vi "Gestione sensori.vi"() -> ()   [LabVIEW 2019]
uses:
  <vilib>/Utility/miscctls.llb/LVRowAndColumnTypeDef.ctl
  <vilib>/Analysis/6fits.llb/Curve Fitting Criteria.ctl
  BenchSelector.vi
  <vilib>/Utility/file.llb/Read Delimited Spreadsheet (string).vi
  Global ingressi analogici.vi
  <vilib>/Analysis/polynomials.llb/Polynomial Plot (Range).vi
  <vilib>/Analysis/1siggen.llb/Ramp Pattern by Delta.vi
  <vilib>/Utility/file.llb/Write Delimited Spreadsheet (string).vi
  <vilib>/Analysis/NI_AALPro.lvlib
  <vilib>/gmath/NI_Gmath.lvlib
  <vilib>/Analysis/NI_AALBase.lvlib
panel:
  out "Row":i32
  out "Input":string[][](array[string])
  out "riga sensore da modificare":string
  out "nome e desc sensore da modificare":string
  out "all rows":string[][](array[string])
  in  "LISTA SENSORI ASSOCIATI":i32(listbox)
  out "Edit Position":T1
  in  "stop":bool
  in  "Unità di Misura":T2
  in  "Tab Control":T3(tab)
  in  "Salva modifica sensore":bool
  in  "SENSORE SELEZIONATO":T4
  in  "modifica sensore":bool
  in  "aggiungi nuovo sensore":bool
  in  "NUOVO SENSORE":T4 {"AI_max" min=0.0}
  in  "carica lista sensori":bool
  in  "Salva lista sensori":bool
  in  "ELIMINA SENSORE":bool
  in  "LISTA SENSORI 2":i32(listbox) caption="LISTA SENSORI"
  in  "MANAGER FUNZIONE CORRETTRICE":bool
  out "MASCHERA 2":bool
  in  "Cluster Funzione correttrice":T5 caption="MANAGER FUNZIONI CORRETTRICI PER LA CATENA INGRESSO+SENSORE"
  out "MASCHERA":bool
  in  "carica mappatura":bool
  in  "Salva mappatura ingressi sensori":bool
  in  "Elimina sensori ingresso selezionato":bool
  in  "Associa sensore":bool
  in  "LISTA SENSORI":i32(listbox) caption="LISTA SENSORI DISPONIBILI"
  in  "MAPPATURA":string[][](table)
  in  "LISTA INGRESSI 3":i32(listbox) caption="LISTA INGRESSI IMPIANTO"
  in  "elimina riga 25":bool
  in  "elimina riga 24":bool
  in  "elimina riga 23":bool
  in  "elimina riga 22":bool
  in  "elimina riga 21":bool
  in  "LINEA 5 - COPPIA":i32(listbox)
  in  "LINEA 4 - COPPIA":i32(listbox)
  in  "LINEA 3 - COPPIA":i32(listbox)
  in  "LINEA 2 - COPPIA":i32(listbox)
  in  "LINEA 1 - COPPIA":i32(listbox)
  in  "elimina riga 20":bool
  in  "elimina riga 19":bool
  in  "elimina riga 18":bool
  in  "elimina riga 17":bool
  in  "elimina riga 16":bool
  in  "LINEA 5 - PRESSIONE PREMISTOPPA":i32(listbox)
  in  "LINEA 4 - PRESSIONE PREMISTOPPA":i32(listbox)
  in  "LINEA 3 - PRESSIONE PREMISTOPPA":i32(listbox)
  in  "LINEA 2 - PRESSIONE PREMISTOPPA":i32(listbox)
  in  "LINEA 1 - PRESSIONE PREMISTOPPA":i32(listbox)
  in  "elimina riga 15":bool
  in  "elimina riga 14":bool
  in  "elimina riga 13":bool
  in  "elimina riga 12":bool
  in  "elimina riga 11":bool
  in  "elimina riga 10":bool
  in  "elimina riga 9":bool
  in  "elimina riga 8":bool
  in  "elimina riga 7":bool
  in  "elimina riga 6":bool
  in  "elimina riga 5":bool
  in  "elimina riga 4":bool
  in  "elimina riga 3":bool
  in  "elimina riga 2":bool
  in  "SVUOTA TUTTO MAPPATURA":bool
  in  "LINEA 5 - PORTATA":i32(listbox)
  in  "LINEA 5 - PRESSIONE ASPIRAZIONE":i32(listbox)
  in  "LINEA 5 - PRESSIONE MANDATA":i32(listbox)
  in  "LINEA 4 - PORTATA":i32(listbox)
  in  "LINEA 4 - PRESSIONE ASPIRAZIONE":i32(listbox)
  in  "LINEA 4 - PRESSIONE MANDATA":i32(listbox)
  in  "carica assoc ingressi- linee":bool
  in  "SALVA ASSOC INGRESSI-LINEE":bool
  in  "LINEA 3 - PORTATA":i32(listbox)
  in  "LINEA 3 - PRESSIONE ASPIRAZIONE":i32(listbox)
  in  "LINEA 3 - PRESSIONE MANDATA":i32(listbox)
  in  "LINEA 2 - PORTATA":i32(listbox)
  in  "LINEA 2 - PRESSIONE ASPIRAZIONE":i32(listbox)
  in  "LINEA 2 - PRESSIONE MANDATA":i32(listbox)
  in  "LINEA 1 - PORTATA":i32(listbox)
  in  "LINEA 1 - PRESSIONE ASPIRAZIONE":i32(listbox)
  in  "LINEA 1 - PRESSIONE MANDATA":i32(listbox)
  in  "LISTA INGRESSI 2":i32(listbox) caption="LISTA INGRESSI"
  in  "elimina riga 1":bool
  in  "Tree":string(tree)
  in  "Cancel Button 2":bool
  in  "Cancel Button":bool
  in  "ASSOCIA 2":bool
  in  "Lista ingressi":i32(listbox)
  in  "ASSOCIA":bool
  in  "Sensori associabili all'ingresso selezionato":i32(listbox)
  # "CLICCA E DIGITA NELLA CELLA DI INTERESSE\nPER IMPOSTARE I VALORI DESIDERATI\nDI RANGE/OFFSET/UM"
  # "CLICCA PER SELEZIONARE \nLA RIGA DI INTERESSE"
  # "MODALITA' DI CONVERSIONE UTILIZZATA PER\nL'INGRESSO+SENSORE SELEZIONATO"
  # "1-SELEZIONA L'INGRESSO DELL'IMPIANTO DESIDERATO DALLA TABELLA \"LISTA INGRESSI IMPIANTO\"\n2-SELEZIONARE IL SENSORE CHE SI VUOLE ASSOCIARE ALL'INGRESSO DALLA TABELLA \"LISTA SENSORI DISPONIBILI\"\n3-CLICCARE \"ASSOCIA SENSORE\"\n4-INSERIRE UM, RANGE ED OFFSET (RELATIVO ALLA CATENA INGRESSO-SENSORE) NELLA TABELLA AFFIANCO\n5-SALVARE LA MAPPATURA CLICCANDO \"SALVA MAPPATURA\""
  # "Inserisci il valore fisico\nimpostato dallo strumento\ndi riferimento"
  # "0=linear fit"
  # "LINEA 1 - VASCA"
  # "LINEA 1 - SERBATOIO"
  # "LINEA 2 - SERBATOIO"
  # "LINEA 3 - SERBATOIO"
  # "LINEA 2 - VASCA"
  # "CLICCA L'INGRESSO DI INTERESSE NELLA \"LISTA INGRESSI\"\nE TRASCINALO NELLA TABELLA OPPORTUNA"
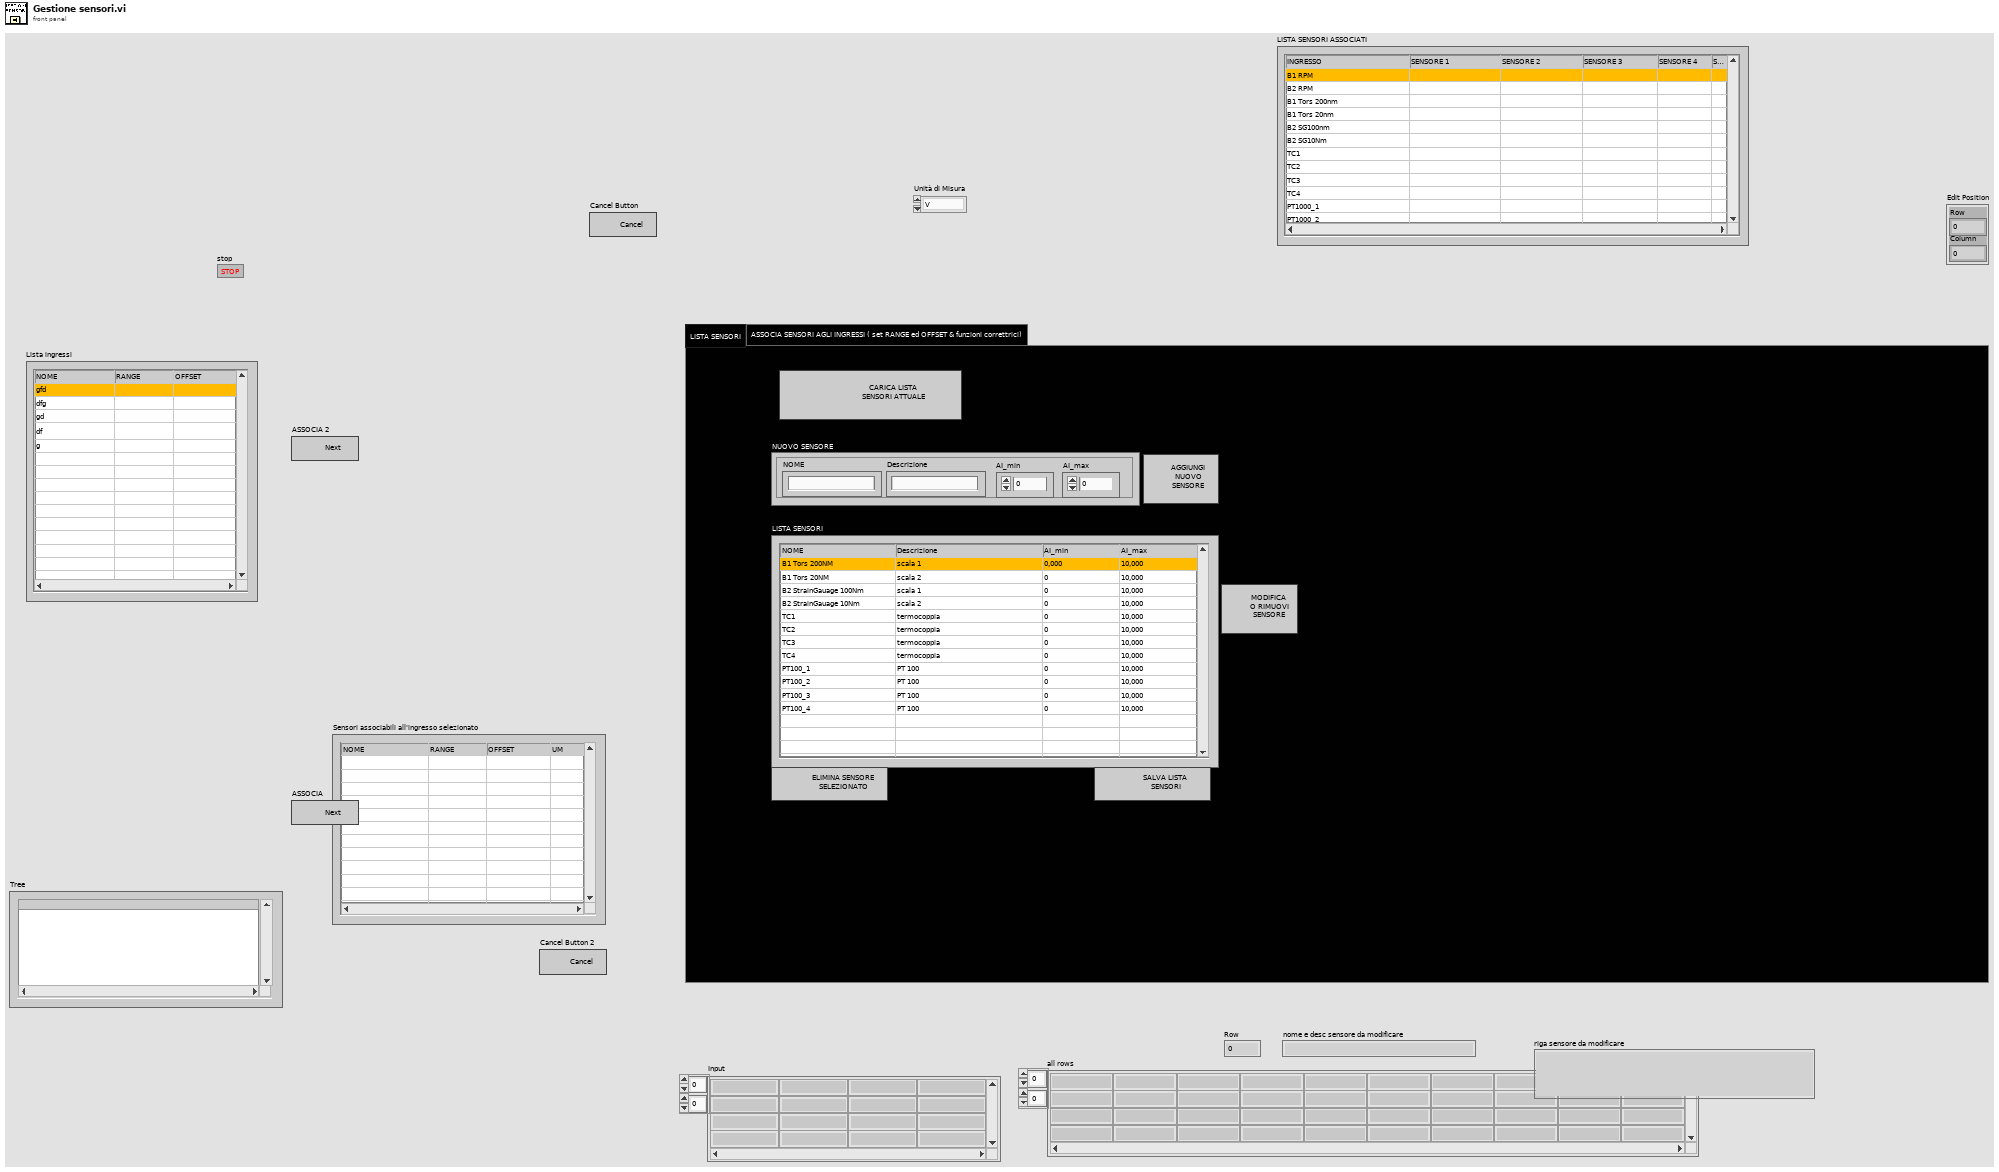
[diagram p1: front panel]
types:
  T1 = typedef "LVRowAndColumnTypeDef.ctl" = cluster{"Row":i32, "Column":i32}
  T2 = typedef "UnitàMisura.ctl" = enum16{"V", "mA", "Bar", "RPM", "m3/s", "m3/min", "m3/h", "l/s", "l/min", "in3/min", "ft3/min", "gpm", "igpm", "igph", "%", "°C", "m", "Nm", "A"}
  T3 = enum32{"LISTA SENSORI", "ASSOCIA SENSORI AGLI INGRESSI ( set RANGE ed OFFSET & funzioni correttrici)", "ASSOCIA GLI INGRESSI ALLE LINEE IDRAULICHE"}
  T4 = cluster{"NOME":string, "Descrizione":string, "AI_min":dbl, "AI_max":dbl}
  T5 = cluster{"Ingresso analogico":dbl, "NOME INGRESSO":string, "NOME SENSORE":string, "DESCRIZIONE":string, "PUNTI FUNZIONE CORRETTRICE":i32, "VALORE FISICO":dbl, "ACQUISISCI PUNTO":bool, "ELIMINA PUNTO":bool, "Valore ingresso analogico":enum32{"Leggi dal campo", "Imposta manualmente"}, "salva funzione correttrice":bool, "Ordine polinomio fit":i16, "Graph":cluster{"Ramp Pattern":dbl[], "P(A)":dbl[]}[], "UM":string, "CHIUDI":bool, "USA FUNZIONE CORRETTRICE?":bool}
  T6 = enum8{"Enabled", "Disabled", "Disabled and Grayed Out"}
  T7 = typedef "NI_AALPro.lvlib/Curve Fitting Criteria.ctl" = u16
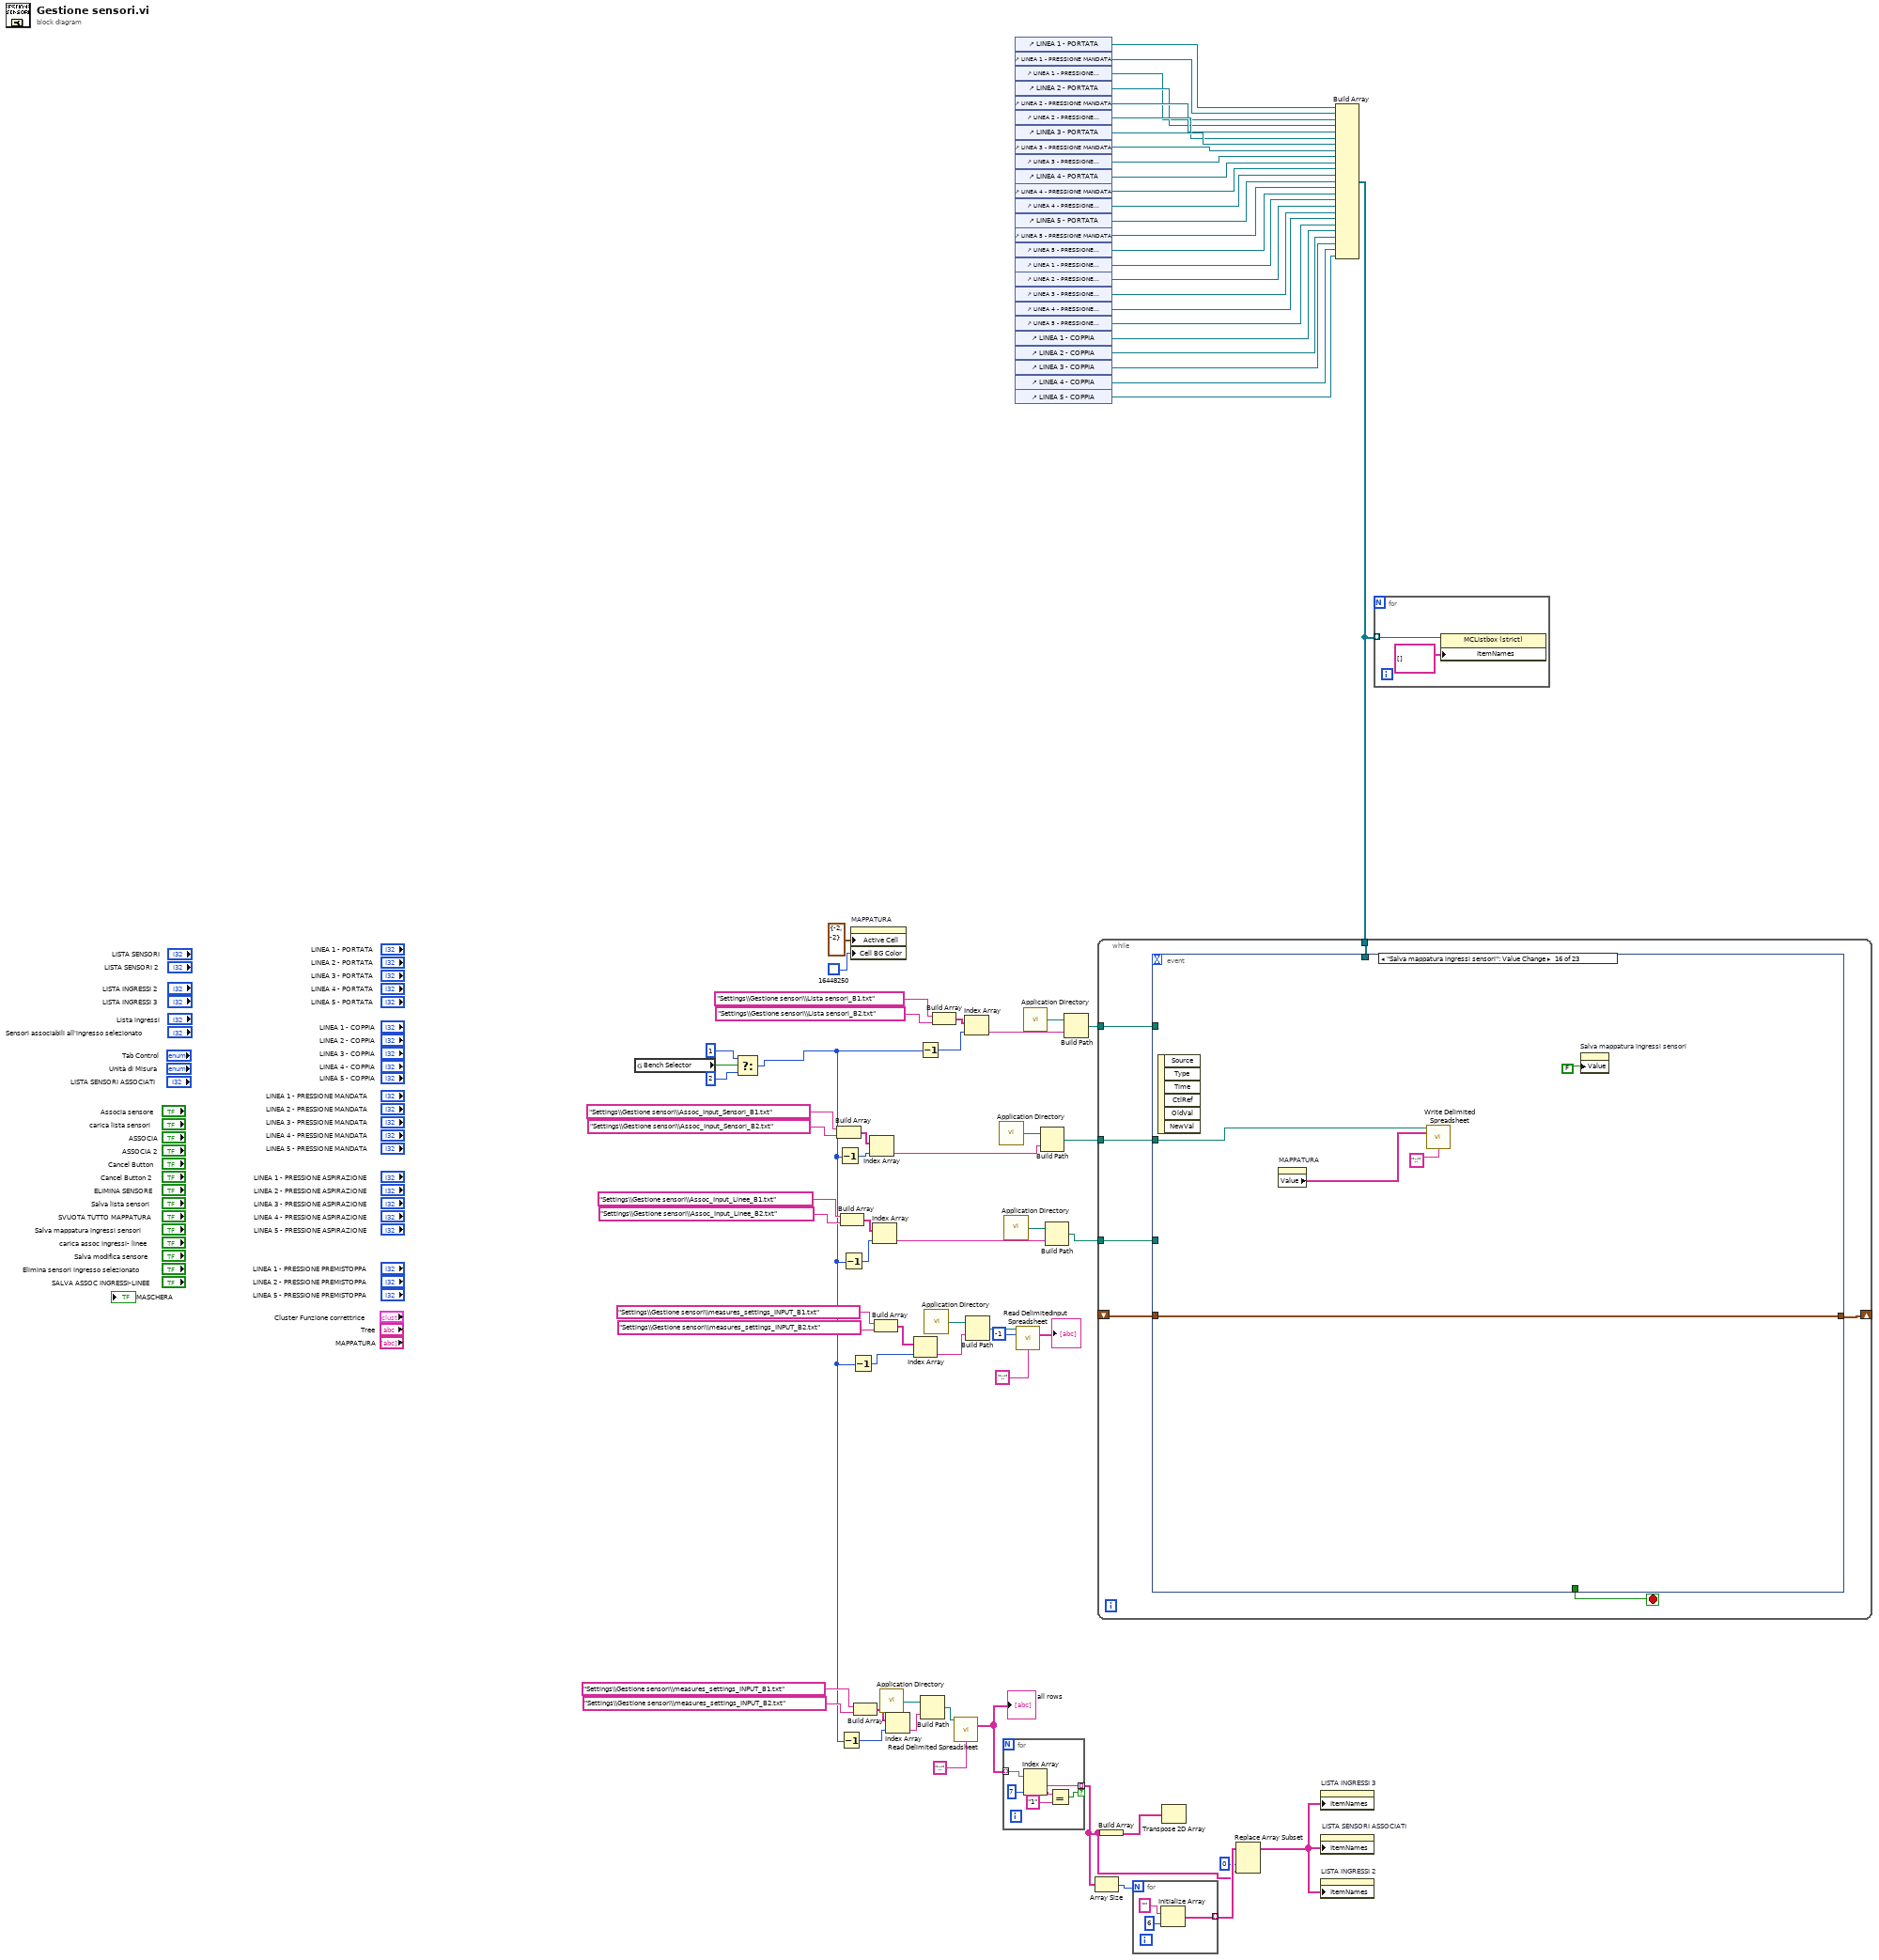
[diagram p0: block diagram]
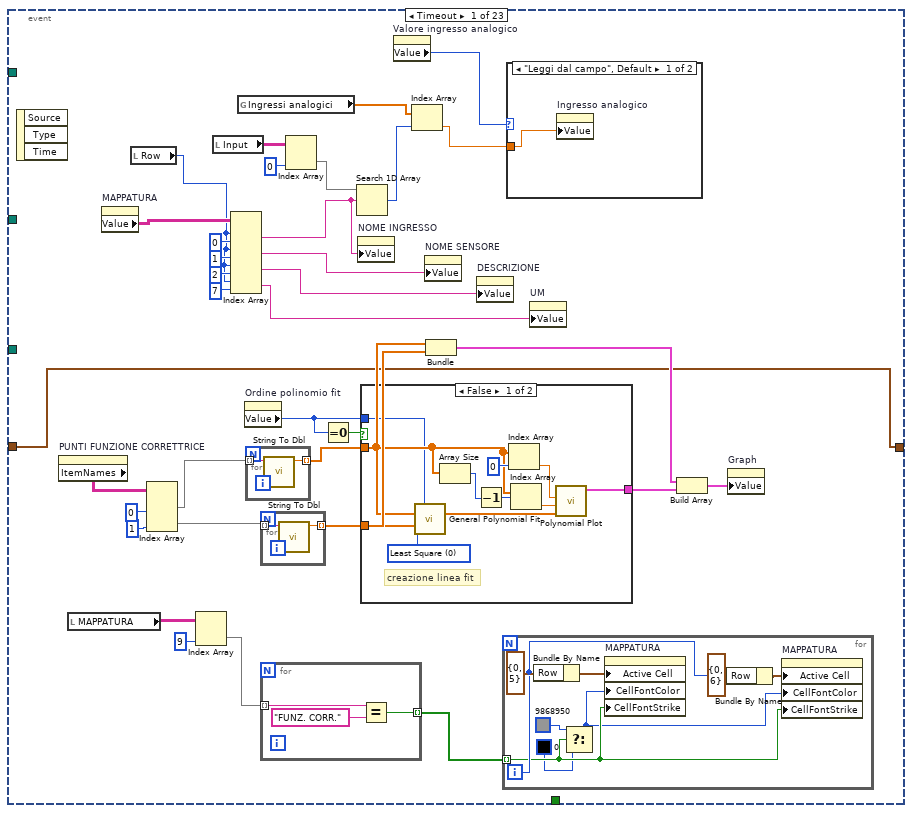
[diagram p2: hidden frame]
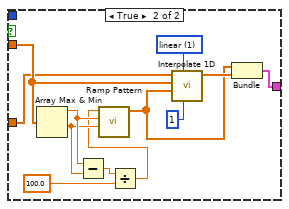
[diagram p3: hidden frame]
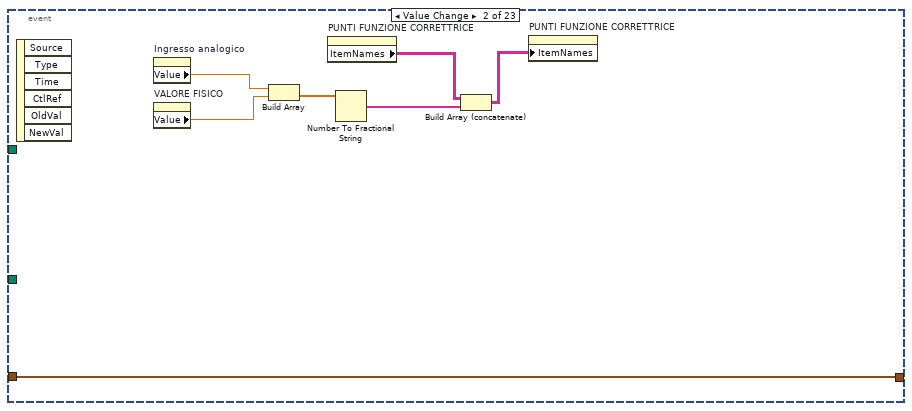
[diagram p5: hidden frame]
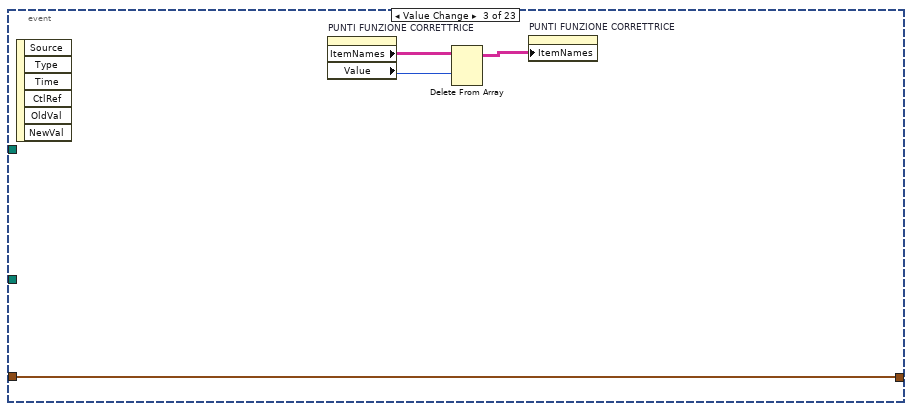
[diagram p6: hidden frame]
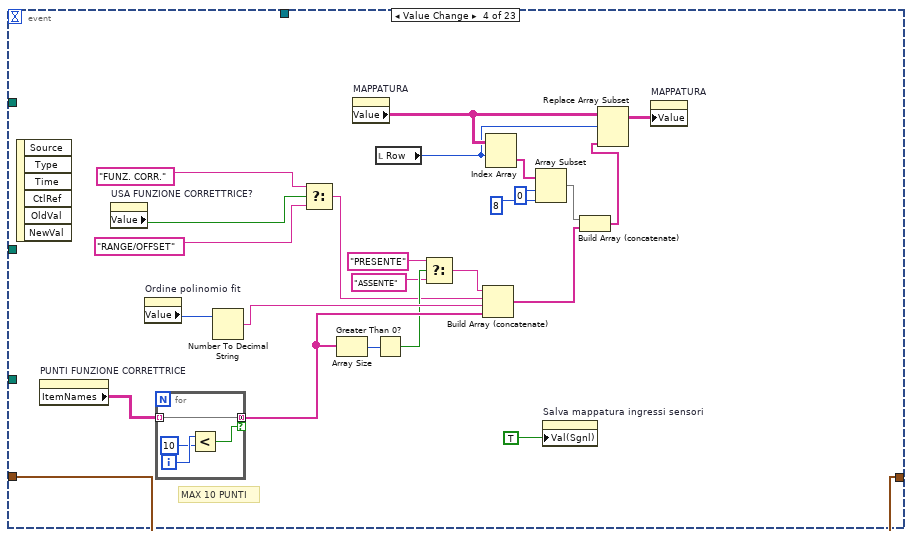
[diagram p7: hidden frame]
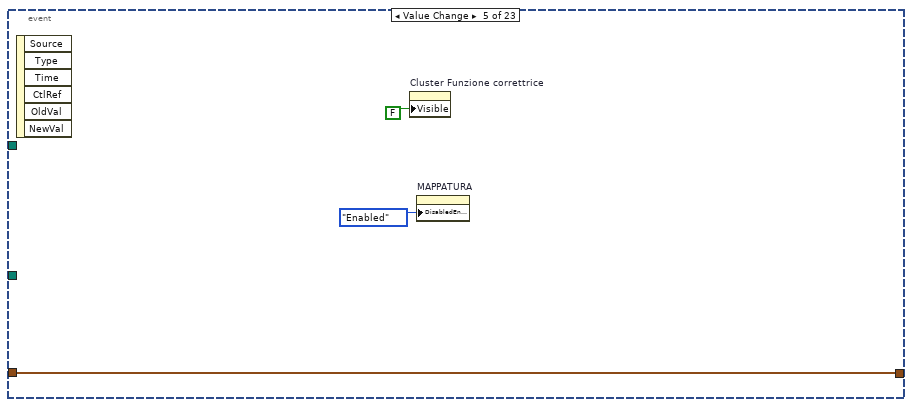
[diagram p8: hidden frame]
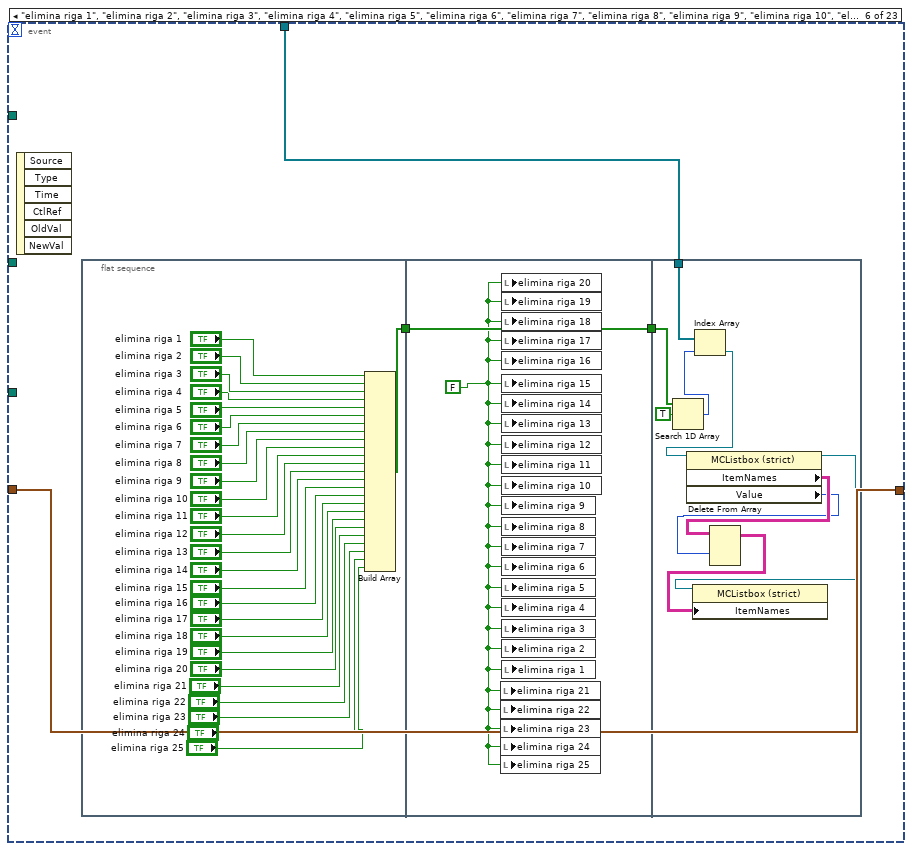
[diagram p9: hidden frame]
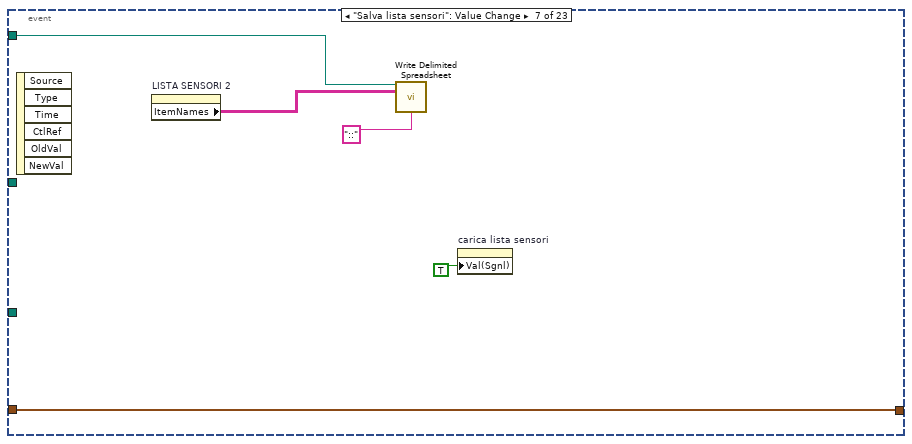
[diagram p10: hidden frame]
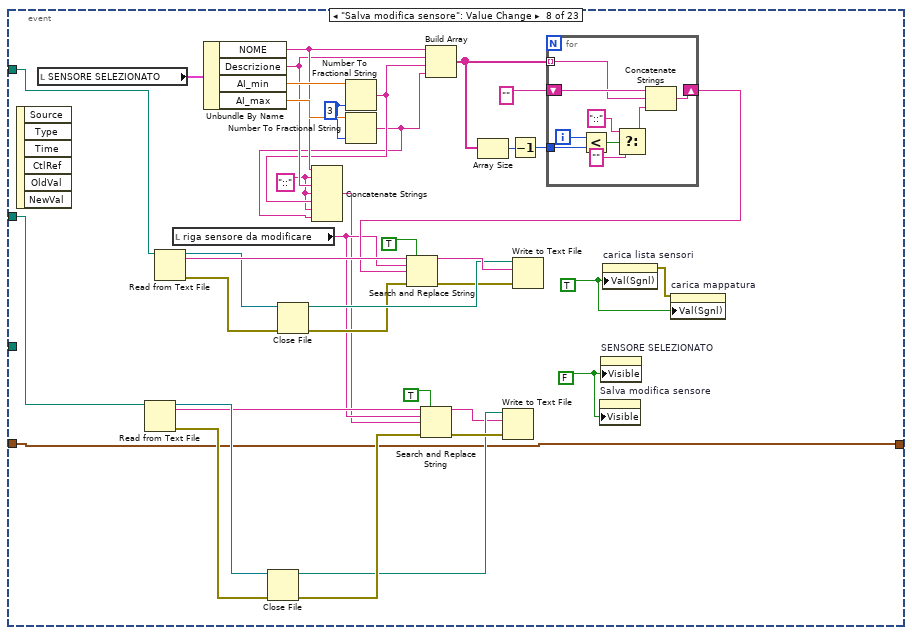
[diagram p11: hidden frame]
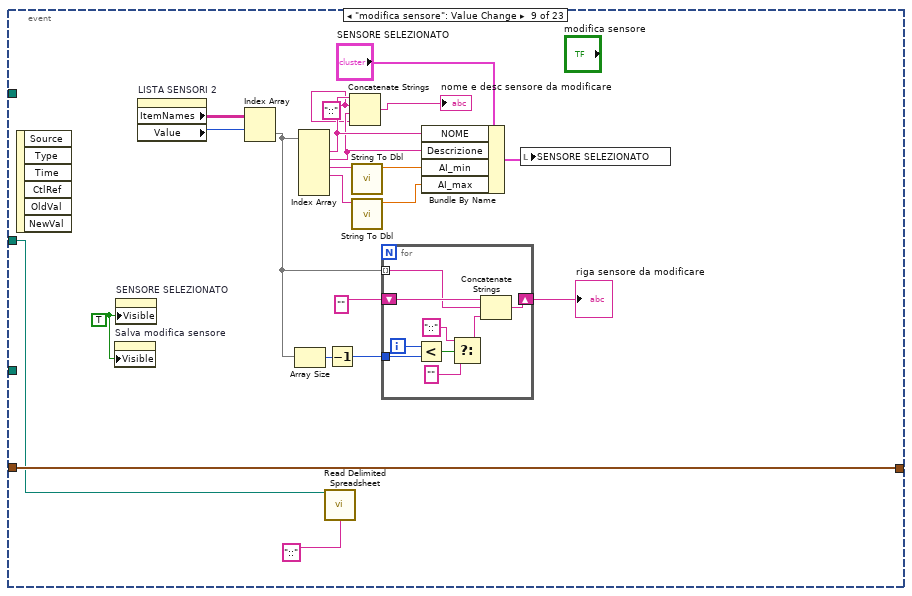
[diagram p12: hidden frame]
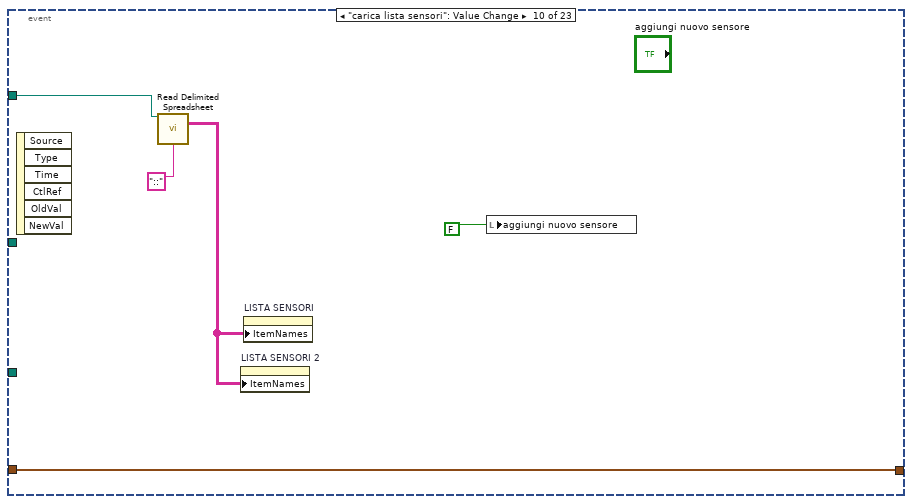
[diagram p13: hidden frame]
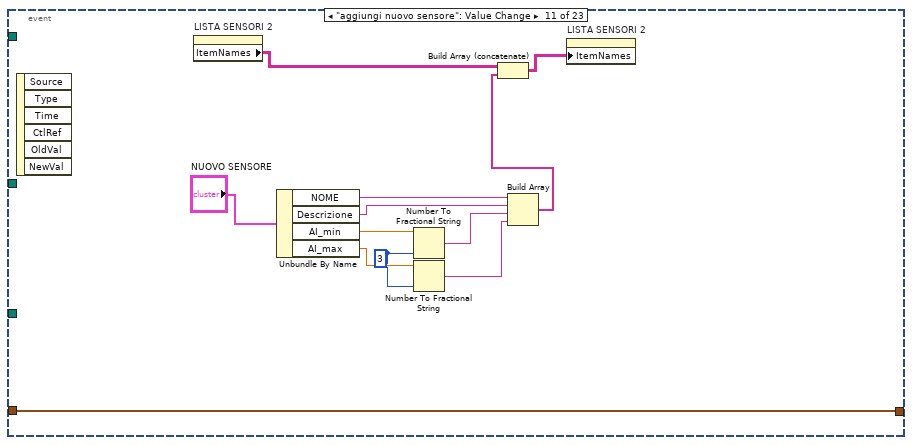
[diagram p14: hidden frame]
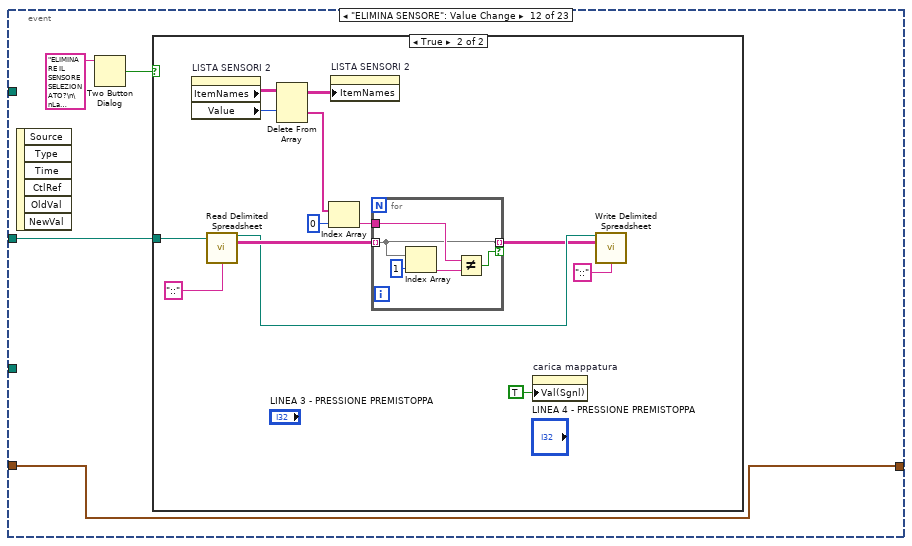
[diagram p15: hidden frame]
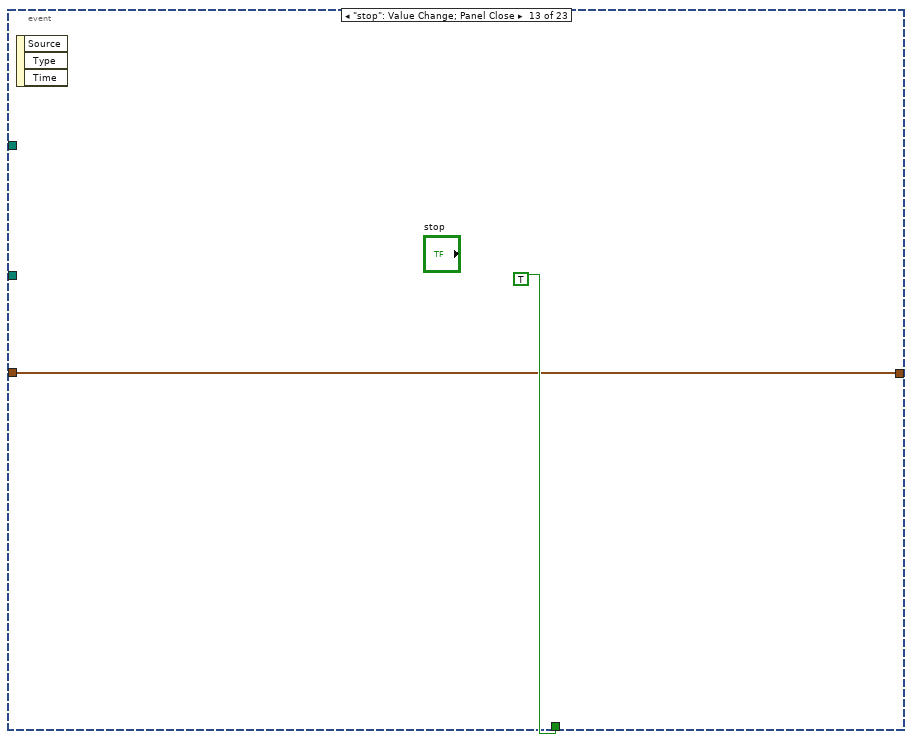
[diagram p17: hidden frame]
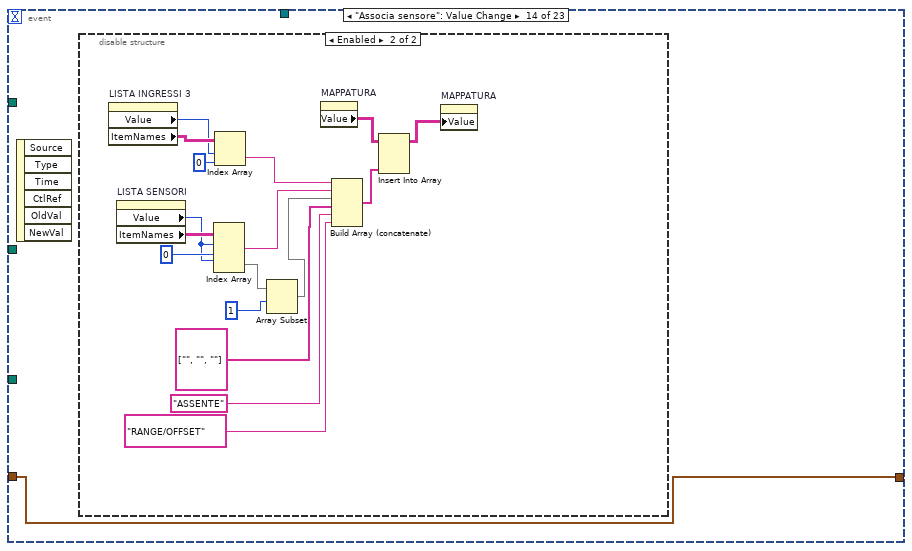
[diagram p18: hidden frame]
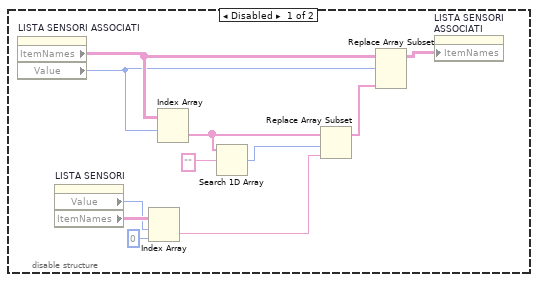
[diagram p19: hidden frame]
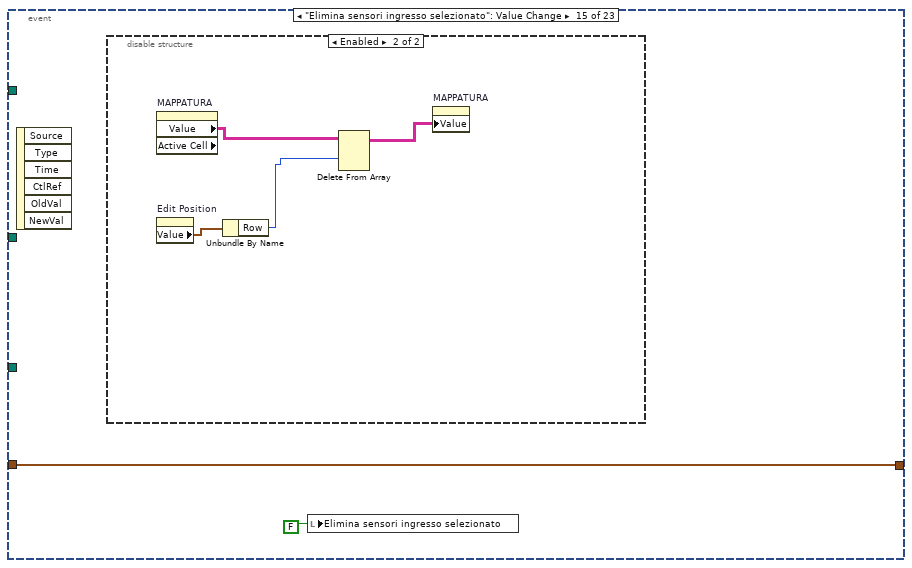
[diagram p20: hidden frame]
diagram:
  n1 = global read "BenchSelector.vi" "Bench Selector"() -> (w1:bool)
  n2 = Select(t=1 ("banco"), s=w1, f=2 ("banco")) -> (s? t:f=w2:i32)
  n3 = Build Array("Settings\\Gestione sensori\\Assoc_Input_Sensori_B1.txt" ("name or relative path"), "Settings\\Gestione sensori\\Assoc_Input_Sensori_B2.txt" ("name or relative path")) -> (w55:string[])
  n4 = Decrement(x=w2) -> (x-1=w54:i32)
  n5 = Decrement(x=w2) -> (x-1=w68:i32)
  n6 = Build Array("Settings\\Gestione sensori\\Assoc_Input_Linee_B1.txt" ("name or relative path"), "Settings\\Gestione sensori\\Assoc_Input_Linee_B2.txt" ("name or relative path")) -> (w49:string[])
  n7 = Decrement(x=w2) -> (x-1=w50:i32)
  n8 = property on="MAPPATURA" class="Tbl (strict)"("Active Cell"=T1 {"Row"=-2, "Column"=-2} ("Active Cell:Active Cell"), "Cell BG Color"=u32 16448250) -> ()  [unwired: 2 in, 2 out]
  n9 = Decrement(x=w2) -> (x-1=w21:i32)
  n10 = Build Array("Settings\\Gestione sensori\\measures_settings_INPUT_B1.txt" ("name or relative path"), "Settings\\Gestione sensori\\measures_settings_INPUT_B2.txt" ("name or relative path")) -> (w69:string[])
  n11 = Index Array(array=w55, index=w54) -> (element=w52:string)
  n12 = Index Array(array=w49, index=w50) -> (element=w45:string)
  n13 = Build Array("Settings\\Gestione sensori\\measures_settings_INPUT_B1.txt" ("name or relative path"), "Settings\\Gestione sensori\\measures_settings_INPUT_B2.txt" ("name or relative path")) -> (w22:string[])
  n14 = call <vilib>:"Application Directory.vi"() -> ("Application Directory"=w67:path)
  n15 = Index Array(array=w69, index=w68) -> (element=w66:string)
  n16 = Index Array(array=w22, index=w21) -> (element=w20:string)
  n17 = Decrement(x=w2) -> (x-1=w77:i32)
  n18 = Build Path(base path=w67, name or relative path=w66) -> (appended path=w65:path)
  n19 = call <vilib>:"Application Directory.vi"() -> ("Application Directory"=w27:path)
  n20 = Build Array("Settings\\Gestione sensori\\Lista sensori_B1.txt" ("name or relative path"), "Settings\\Gestione sensori\\Lista sensori_B2.txt" ("name or relative path")) -> (w76:string[])
  n21 = call-poly <vilib>:"Read Delimited Spreadsheet.vi"("file path (dialog if empty)"=w65, "delimiter (\\t)"="::" ("delimiter (\\t)")) -> ("all rows"=w63:string[][])  [unwired: 8 in, 5 out]
  "all rows" <- w63
  n22 = Index Array(array=w76, index=w77) -> (element=w73:string)
  n23 = Build Path(base path=w27, name or relative path=w20) -> (appended path=w26:path)
  n24 = call <vilib>:"Application Directory.vi"() -> ("Application Directory"=w53:path)
  n25 = for {
    tunnel: w63 -> [w84] mode=indexing
    tunnel: [w81] -> w58 mode=indexing if=w80
    n26 = Index Array(array=w84, index #2=7 ("index")) -> (element #1=w81:string, element #2=w83:string)  [unwired: 1 in]
    n27 = Equal?(x=w83, y="1") -> (x = y?=w80:bool)
  }
  n28 = call <vilib>:"Application Directory.vi"() -> ("Application Directory"=w46:path)
  n29 = control-ref of="LINEA 1 - PORTATA"() -> (w35:refnum<vi>)
  n30 = control-ref of="LINEA 1 - PRESSIONE MANDATA"() -> (w36:refnum<vi>)
  n31 = control-ref of="LINEA 1 - PRESSIONE ASPIRAZIONE"() -> (w37:refnum<vi>)
  n32 = control-ref of="LINEA 2 - PORTATA"() -> (w38:refnum<vi>)
  n33 = control-ref of="LINEA 2 - PRESSIONE MANDATA"() -> (w39:refnum<vi>)
  n34 = control-ref of="LINEA 2 - PRESSIONE ASPIRAZIONE"() -> (w40:refnum<vi>)
  n35 = control-ref of="LINEA 3 - PORTATA"() -> (w41:refnum<vi>)
  n36 = control-ref of="LINEA 3 - PRESSIONE MANDATA"() -> (w42:refnum<vi>)
  n37 = control-ref of="LINEA 3 - PRESSIONE ASPIRAZIONE"() -> (w43:refnum<vi>)
  n38 = control-ref of="LINEA 4 - PORTATA"() -> (w33:refnum<vi>)
  n39 = control-ref of="LINEA 4 - PRESSIONE MANDATA"() -> (w32:refnum<vi>)
  n40 = control-ref of="LINEA 4 - PRESSIONE ASPIRAZIONE"() -> (w31:refnum<vi>)
  n41 = control-ref of="LINEA 5 - PORTATA"() -> (w30:refnum<vi>)
  n42 = control-ref of="LINEA 5 - PRESSIONE MANDATA"() -> (w29:refnum<vi>)
  n43 = control-ref of="LINEA 5 - PRESSIONE ASPIRAZIONE"() -> (w28:refnum<vi>)
  n44 = control-ref of="LINEA 1 - PRESSIONE PREMISTOPPA"() -> (w14:refnum<vi>)
  n45 = control-ref of="LINEA 2 - PRESSIONE PREMISTOPPA"() -> (w13:refnum<vi>)
  n46 = control-ref of="LINEA 3 - PRESSIONE PREMISTOPPA"() -> (w12:refnum<vi>)
  n47 = control-ref of="LINEA 4 - PRESSIONE PREMISTOPPA"() -> (w11:refnum<vi>)
  n48 = control-ref of="LINEA 5 - PRESSIONE PREMISTOPPA"() -> (w10:refnum<vi>)
  n49 = control-ref of="LINEA 1 - COPPIA"() -> (w9:refnum<vi>)
  n50 = control-ref of="LINEA 2 - COPPIA"() -> (w8:refnum<vi>)
  n51 = control-ref of="LINEA 3 - COPPIA"() -> (w7:refnum<vi>)
  n52 = control-ref of="LINEA 4 - COPPIA"() -> (w6:refnum<vi>)
  n53 = control-ref of="LINEA 5 - COPPIA"() -> (w5:refnum<vi>)
  n54 = call-poly <vilib>:"Read Delimited Spreadsheet.vi"("file path (dialog if empty)"=w26, "number of rows (all:-1)"=-1, "delimiter (\\t)"="::" ("delimiter (\\t)")) -> ("all rows"=→"Input":string[][])  [unwired: 7 in, 5 out]
  n55 = call <vilib>:"Application Directory.vi"() -> ("Application Directory"=w78:path)
  n56 = Build Path(base path=w53, name or relative path=w52) -> (appended path=w51:path)
  n57 = Build Path(base path=w46, name or relative path=w45) -> (appended path=w44:path)
  n58 = Build Path(base path=w78, name or relative path=w73) -> (appended path=w72:path)
  n59 = Array Size(array=w58) -> (size(s)=w61:i32)
  n60 = Build Array(w58) -> (w62:string[][])
  n61 = for {
    N: w61 -> [_]
    tunnel: [w85] -> w60 mode=indexing
    n62 = Initialize Array("", 6 ("dimension size")) -> (w85:string[])
  }
  n63 = Transpose 2D Array(2D array=w62) -> ()  [unwired: 1 out]
  n64 = Replace Array Subset(array=w60, new element=w58, index (col)=0 ("disabled index (col)")) -> (w34:string[][])  [unwired: 1 in]
  n65 = property on="LISTA INGRESSI 3" class="MCListbox (strict)"("ItemNames"=w34) -> ()  [unwired: 2 in, 2 out]
  n66 = property on="LISTA SENSORI ASSOCIATI" class="MCListbox (strict)"("ItemNames"=w34) -> ()  [unwired: 2 in, 2 out]
  n67 = property on="LISTA INGRESSI 2" class="MCListbox (strict)"("ItemNames"=w34) -> ()  [unwired: 2 in, 2 out]
  n68 = Build Array(w35, w36, w37, w38, w39, w40, w41, w42, w43, w33, w32, w31, w30, w29, w28, w14, w13, w12, w11, w10, w9, w8, w7, w6, w5) -> (w17:refnum<vi>[])
  n69 = while {
    tunnel: w72 -> [w94]
    tunnel: w51 -> [w92]
    tunnel: w44 -> [w91]
    tunnel: w17 -> [w90]
    shift-right: [w89] -> _
    shift-left: _ -> [w88]
    stop <- w93 stop-if-true
    n70 = event shown="[15] \"Salva mappatura ingressi sensori\": Value Change" {
      selector: _ -> [_ _ _ _ _ _ _ _ _ _ _ _ _ _ _ _ _ _ _ _ _ _ _]
      dyn-events: _ -> [_ _ _ _ _ _ _ _ _ _ _ _ _ _ _ _ _ _ _ _ _ _ _]
      timeout: _ -> [_ _ _ _ _ _ _ _ _ _ _ _ _ _ _ _ _ _ _ _ _ _ _]
      tunnel: w94 -> [_ _ _ _ _ _ w255 w287 _ w338 _ _ _ _ _ _ _ _ _ _ _ _ _]
      tunnel: [_ _ _ _ _ _ _ _ _ _ _ _ TRUE _ _ _ _ _ _ _ _ _ _] -> w93
      tunnel: w92 -> [_ _ _ _ _ _ _ w268 w304 _ _ w352 _ _ _ w421 w427 _ _ _ _ _ _]
      tunnel: w91 -> [_ _ _ _ _ _ _ _ _ _ _ _ _ _ _ _ _ _ _ _ w557 w602 _]
      tunnel: w90 -> [_ _ _ _ _ w214 _ _ _ _ _ _ _ _ _ _ _ _ _ _ _ _ _]
      tunnel: [w101 w169 w176 w184 w208 w211 w252 w263 w306 w334 w339 w351 w373 w375 w405 w418 w423 w448 w495 w523 w550 w600 w637] -> w89
      tunnel: w88 -> [w101 w169 w176 w184 w208 w211 w252 w263 w306 w334 w339 w351 w373 w375 w405 w418 w423 w448 w495 w522 w550 w600 w637]
      event Timeout {
        n71 = event-data() -> ()  [unwired: 1 in, 3 out]
        n72 = property on="PUNTI FUNZIONE CORRETTRICE" class="MCListbox (strict)"() -> ("ItemNames"=w120:string[][])  [unwired: 2 in, 2 out]
        n73 = local read "MAPPATURA"() -> (w100:string[][])
        n74 = property on="MAPPATURA" class="Tbl (strict)"() -> ("Value"=w110:string[][])  [unwired: 2 in, 2 out]
        n75 = local read "Row"() -> (w102:i32)
        n76 = Index Array(array=w120, index (col) #1=0 ("disabled index (col)"), index (col) #2=1 ("index (col)")) -> (element #1=w118:string[], element #2=w117:string[])  [unwired: 2 in]
        n77 = Index Array(array=w100, index (col)=9 ("disabled index (col)")) -> (element=w98:string[])  [unwired: 1 in]
        n78 = local read "Input"() -> (w126:string[][])
        n79 = Index Array(array=w110, index (row) #1=w102, index (col) #1=0 ("disabled index (col)"), index (row) #2=w102, index (col) #2=1 ("disabled index (col)"), index (row) #3=w102, index (col) #3=2 ("disabled index (col)"), index (row) #4=w102, index (col) #4=7 ("disabled index (col)")) -> (element #1=w109:string, element #2=w106:string, element #3=w105:string, element #4=w103:string)
        n80 = global read "Global ingressi analogici.vi" "Ingressi analogici"() -> (w128:dbl[])
        n81 = property on="Ordine polinomio fit" class="DigNum (strict)"() -> ("Value"=w96:i16)  [unwired: 2 in, 2 out]
        n82 = for {
          tunnel: w118 -> [w167] mode=indexing
          tunnel: [w166] -> w114 mode=indexing
          n83 = call "String To Dbl.vi"("String"=w167) -> ("Numeric"=w166:dbl)  [unwired: 10 in]
        }
        n84 = for {
          tunnel: w117 -> [w165] mode=indexing
          tunnel: [w164] -> w113 mode=indexing
          n85 = call "String To Dbl.vi"("String"=w165) -> ("Numeric"=w164:dbl)  [unwired: 10 in]
        }
        n86 = for {
          tunnel: w98 -> [w163] mode=indexing
          tunnel: [w161] -> w97 mode=indexing
          n87 = Equal?(x=w163, y="FUNZ. CORR.") -> (x = y?=w161:bool)
        }
        n88 = Index Array(array=w126, index (col)=0 ("disabled index (col)")) -> (element=w124:string[])  [unwired: 1 in]
        n89 = Equal To 0?(x=w96) -> (x = 0?=w95:bool)
        n90 = Search 1D Array(1D array=w124, element=w109) -> (index of element=w123:i32)  [unwired: 1 in]
        n91 = property on="NOME INGRESSO" class="Str"("Value"=w109) -> ()  [unwired: 2 in, 2 out]
        n92 = case shown="False" w95 {
          tunnel: [w137 w143] -> w116
          tunnel: w114 -> [w131 w141]
          tunnel: w113 -> [w130 w140]
          tunnel: w96 -> [w129 _]
          frame False {
            w132 = T7 0 items=["Least Square", "Least Absolute Residual", "Bisquare"] ("method")
            # "creazione linea fit"
            n93 = call <vilib>:"General Polynomial Fit.vi"("Y"=w130, "polynomial order"=w129, "X"=w131, "method"=w132) -> ("Polynomial Coefficients"=w134:dbl[])  [unwired: 8 in, 3 out]
            n94 = Array Size(array=w131) -> (size(s)=w139:i32)
            n95 = Decrement(x=w139) -> (x-1=w138:i32)
            n96 = Index Array(array=w131, index=0) -> (element=w135:dbl)
            n97 = Index Array(array=w131, index=w138) -> (element=w136:dbl)
            n98 = call-poly <vilib>:"Polynomial Plot.vi"("P(x)"=w134, "end"=w136, "start"=w135) -> ("polynomial plot"=w137:cluster{"Ramp Pattern":dbl[], "P(A)":dbl[]})  [unwired: 7 in, 1 out]
          }
          frame True {
            w151 = 1 items=["nearest", "linear", "spline", "cubic Hermite", "Lagrange"] ("method")
            n99 = Array Max & Min(array=w141) -> (max value=w149:dbl, min value=w148:dbl)  [unwired: 2 out]
            n100 = Subtract(x=w149, y=w148) -> (x-y=w147:dbl)
            n101 = Divide(x=w147, y=100.0) -> (x/y=w145:dbl)
            n102 = call-poly <vilib>:"Ramp Pattern.vi"("start"=w148, "end"=w149, "delta"=w145) -> ("Ramp Pattern"=w142:dbl[])  [unwired: 6 in, 2 out]
            n103 = call <vilib>:"Interpolate 1D.vi"("ntimes"=1, "method"=w151, "xi"=w142, "X"=w141, "Y"=w140) -> ("yi"=w144:dbl[])  [unwired: 4 in, 2 out]
            n104 = Bundle("Ramp Pattern"=w142, "yi"=w144) -> (w143:cluster{"Ramp Pattern":dbl[], "yi":dbl[]})  [unwired: 1 in]
          }
        }
        n105 = property on="Valore ingresso analogico" class="RadioBtnsControl (strict)"() -> ("Value"=w122:enum32{"Leggi dal campo", "Imposta manualmente"})  [unwired: 2 in, 2 out]
        n106 = Index Array(array=w128, index=w123) -> (element=w121:dbl)
        n107 = property on="NOME SENSORE" class="Str"("Value"=w106) -> ()  [unwired: 2 in, 2 out]
        n108 = Bundle(w114, w113) -> (w115:cluster{dbl[], dbl[]})  [unwired: 1 in]
        n109 = property on="DESCRIZIONE" class="Str"("Value"=w105) -> ()  [unwired: 2 in, 2 out]
        n110 = for {
          tunnel: w97 -> [w155] mode=indexing
          i -> [w156]
          n111 = Bundle By Name(cluster=T1 {"Row"=0, "Column"=5} ("Active Cell:Active Cell"), "Row"=w156) -> (w159:T1)
          n112 = Select(t=u32 9868950, s=w155, f=u32 0) -> (s? t:f=w152:u32)
          n113 = property on="MAPPATURA" class="Tbl (strict)"("Active Cell"=w159, "CellFontColor"=w152, "CellFontStrike"=w155) -> ()  [unwired: 2 in, 2 out]
          n114 = Bundle By Name(cluster=T1 {"Row"=0, "Column"=6} ("Active Cell:Active Cell"), "Row"=w156) -> (w158:T1)
          n115 = property on="MAPPATURA" class="Tbl (strict)"("Active Cell"=w158, "CellFontColor"=w152, "CellFontStrike"=w155) -> ()  [unwired: 2 in, 2 out]
        }
        n116 = case shown="\"Leggi dal campo\", Default" w122 {
          tunnel: w121 -> [w168 _]
          frame "Leggi dal campo", Default {
            n117 = property on="Ingresso analogico" class="DigNum (strict)"("Value"=w168) -> ()  [unwired: 2 in, 2 out]
          }
          frame "Imposta manualmente" {
          }
        }
        n118 = property on="UM" class="Str"("Value"=w103) -> ()  [unwired: 2 in, 2 out]
        n119 = Build Array(w115, w116) -> (w112:cluster{"Ramp Pattern":dbl[], "yi":dbl[]}[])
        n120 = property on="Graph" class="XYGraph (strict)"("Value"=w112) -> ()  [unwired: 2 in, 2 out]
      }
      event "Cluster Funzione correttrice.ACQUISISCI PUNTO": Value Change {
        n121 = event-data() -> ()  [unwired: 1 in, 6 out]
        n122 = property on="Ingresso analogico" class="DigNum (strict)"() -> ("Value"=w175:dbl)  [unwired: 2 in, 2 out]
        n123 = property on="VALORE FISICO" class="DigNum (strict)"() -> ("Value"=w174:dbl)  [unwired: 2 in, 2 out]
        n124 = Build Array(w175, w174) -> (w173:dbl[])
        n125 = property on="PUNTI FUNZIONE CORRETTRICE" class="MCListbox (strict)"() -> ("ItemNames"=w172:string[][])  [unwired: 2 in, 2 out]
        n126 = Number To Fractional String(number=w173) -> (F-format string=w170:string[])  [unwired: 3 in]
        n127 = Build Array (concatenate)(w172, w170) -> (w171:string[][])
        n128 = property on="PUNTI FUNZIONE CORRETTRICE" class="MCListbox (strict)"("ItemNames"=w171) -> ()  [unwired: 2 in, 2 out]
      }
      event "Cluster Funzione correttrice.ELIMINA PUNTO": Value Change {
        n129 = event-data() -> ()  [unwired: 1 in, 6 out]
        n130 = property on="PUNTI FUNZIONE CORRETTRICE" class="MCListbox (strict)"() -> ("ItemNames"=w179:string[][], "Value"=w177:i32)  [unwired: 2 in, 2 out]
        n131 = Delete From Array(array=w179, index (row)=w177) -> (array with subset deleted=w178:string[][])  [unwired: 2 in, 1 out]
        n132 = property on="PUNTI FUNZIONE CORRETTRICE" class="MCListbox (strict)"("ItemNames"=w178) -> ()  [unwired: 2 in, 2 out]
      }
      event "Cluster Funzione correttrice.salva funzione correttrice": Value Change {
        # "MAX 10 PUNTI"
        n133 = event-data() -> ()  [unwired: 1 in, 6 out]
        n134 = property on="PUNTI FUNZIONE CORRETTRICE" class="MCListbox (strict)"() -> ("ItemNames"=w203:string[][])  [unwired: 2 in, 2 out]
        n135 = property on="USA FUNZIONE CORRETTRICE?" class="Bool (strict)"() -> ("Value"=w183:bool)  [unwired: 2 in, 2 out]
        n136 = property on="Ordine polinomio fit" class="DigNum (strict)"() -> ("Value"=w202:i16)  [unwired: 2 in, 2 out]
        n137 = for {
          tunnel: w203 -> [w207] mode=indexing
          tunnel: [w207] -> w200 mode=concatenating if=w204
          i -> [w206]
          n138 = Less?(x=w206, y=10) -> (x < y?=w204:bool)
        }
        n139 = Number To Decimal String(number=w202) -> (decimal integer string=w201:string)  [unwired: 1 in]
        n140 = Select(t="FUNZ. CORR.", s=w183, f="RANGE/OFFSET") -> (s? t:f=w180:string)
        n141 = Array Size(array=w200) -> (size(s)=w199:i32)
        n142 = property on="MAPPATURA" class="Tbl (strict)"() -> ("Value"=w189:string[][])  [unwired: 2 in, 2 out]
        n143 = Greater Than 0?(x=w199) -> (x > 0?=w198:bool)
        n144 = local read "Row"() -> (w186:i32)
        n145 = Select(t="PRESENTE", s=w198, f="ASSENTE") -> (s? t:f=w196:string)
        n146 = Build Array (concatenate)(w196, w180, w201, w200) -> (w190:string[])
        n147 = Index Array(array=w189, index (row)=w186) -> (element=w194:string[])  [unwired: 1 in]
        n148 = Array Subset(array=w194, index=0, length=8) -> (w191:string[])
        n149 = property on="Salva mappatura ingressi sensori" class="Bool (strict)"("Val(Sgnl)"=TRUE) -> ()  [unwired: 2 in, 2 out]
        n150 = Build Array (concatenate)(w191, w190) -> (w187:string[])
        n151 = Replace Array Subset(array=w189, new element=w187, index (row)=w186) -> (w188:string[][])  [unwired: 1 in]
        n152 = property on="MAPPATURA" class="Tbl (strict)"("Value"=w188) -> ()  [unwired: 2 in, 2 out]
      }
      event "Cluster Funzione correttrice.CHIUDI": Value Change {
        n153 = event-data() -> ()  [unwired: 1 in, 6 out]
        n154 = property on="Cluster Funzione correttrice" class="Clust"("Visible"=FALSE) -> ()  [unwired: 2 in, 2 out]
        n155 = property on="MAPPATURA" class="Tbl (strict)"("DisabledEnum"=T6."Enabled" ("Disabled")) -> ()  [unwired: 2 in, 2 out]
      }
      event "elimina riga 1", "elimina riga 2", "elimina riga 3", "elimina riga 4", "elimina riga 5", "elimina riga 6", "elimina riga 7", "elimina riga 8", "elimina riga 9", "elimina riga 10", "elimina riga 11", "elimina riga 12", "elimina riga 13", "elimina riga 14", "elimina riga 15", "elimina riga 16", "elimina riga 17", "elimina riga 18", "elimina riga 19", "elimina riga 20", "elimina riga 21", "elimina riga 22", "elimina riga 23", "elimina riga 24", "elimina riga 25": Value Change {
        n156 = event-data() -> ()  [unwired: 1 in, 6 out]
        n157 = flat-sequence {
          tunnel: [w225] -> w213
          tunnel: w213 -> [w242]
          tunnel: [w242] -> w212
          tunnel: w214 -> [w251]
          tunnel: w212 -> [w250]
          frame #0 {
            n158 = Build Array("elimina riga 1", "elimina riga 2", "elimina riga 3", "elimina riga 4", "elimina riga 5", "elimina riga 6", "elimina riga 7", "elimina riga 8", "elimina riga 9", "elimina riga 10", "elimina riga 11", "elimina riga 12", "elimina riga 13", "elimina riga 14", "elimina riga 15", "elimina riga 16", "elimina riga 17", "elimina riga 18", "elimina riga 19", "elimina riga 20", "elimina riga 21", "elimina riga 22", "elimina riga 23", "elimina riga 24", "elimina riga 25") -> (w225:bool[])
          }
          frame #1 {
            w241 = FALSE
            n159 = local write "elimina riga 21"(w241) -> ()
            n160 = local write "elimina riga 22"(w241) -> ()
            n161 = local write "elimina riga 23"(w241) -> ()
            n162 = local write "elimina riga 24"(w241) -> ()
            n163 = local write "elimina riga 25"(w241) -> ()
            n164 = local write "elimina riga 20"(w241) -> ()
            n165 = local write "elimina riga 19"(w241) -> ()
            n166 = local write "elimina riga 18"(w241) -> ()
            n167 = local write "elimina riga 17"(w241) -> ()
            n168 = local write "elimina riga 16"(w241) -> ()
            n169 = local write "elimina riga 15"(w241) -> ()
            n170 = local write "elimina riga 14"(w241) -> ()
            n171 = local write "elimina riga 13"(w241) -> ()
            n172 = local write "elimina riga 12"(w241) -> ()
            n173 = local write "elimina riga 11"(w241) -> ()
            n174 = local write "elimina riga 10"(w241) -> ()
            n175 = local write "elimina riga 9"(w241) -> ()
            n176 = local write "elimina riga 8"(w241) -> ()
            n177 = local write "elimina riga 7"(w241) -> ()
            n178 = local write "elimina riga 6"(w241) -> ()
            n179 = local write "elimina riga 5"(w241) -> ()
            n180 = local write "elimina riga 4"(w241) -> ()
            n181 = local write "elimina riga 3"(w241) -> ()
            n182 = local write "elimina riga 2"(w241) -> ()
            n183 = local write "elimina riga 1"(w241) -> ()
          }
          frame #2 {
            n184 = Search 1D Array(1D array=w250, element=TRUE) -> (index of element=w248:i32)  [unwired: 1 in]
            n185 = Index Array(array=w251, index=w248) -> (element=w247:refnum<vi>)
            n186 = property class="MCListbox (strict)"(reference=w247) -> (reference out=w244:refnum<vi>, "ItemNames"=w246:string[][], "Value"=w245:i32)  [unwired: 1 in, 1 out]
            n187 = Delete From Array(array=w246, index (row)=w245) -> (array with subset deleted=w243:string[][])  [unwired: 2 in, 1 out]
            n188 = property class="MCListbox (strict)"(reference=w244, "ItemNames"=w243) -> ()  [unwired: 1 in, 2 out]
          }
        }
      }
      event "Salva lista sensori": Value Change {
        n189 = event-data() -> ()  [unwired: 1 in, 6 out]
        n190 = property on="LISTA SENSORI 2" class="MCListbox (strict)"() -> ("ItemNames"=w254:string[][])  [unwired: 2 in, 2 out]
        n191 = call-poly <vilib>:"Write Delimited Spreadsheet.vi"("file path (dialog if empty)"=w255, "2D data"=w254, "delimiter (\\t)"="::" ("delimiter (\\t)")) -> ()  [unwired: 11 in, 2 out]
        n192 = property on="carica lista sensori" class="Bool (strict)"("Val(Sgnl)"=TRUE ("Value (Signaling)")) -> ()  [unwired: 2 in, 2 out]
      }
      event "Salva modifica sensore": Value Change {
        w259 = "::" ("string")
        w266 = TRUE ("Value (Signaling)")
        w277 = FALSE ("Visible")
        w291 = i16 3 ("precision (6)")
        n193 = event-data() -> ()  [unwired: 1 in, 6 out]
        n194 = local read "SENSORE SELEZIONATO"() -> (w294:T4)
        n195 = Read from Text File(file (use dialog)=w268) -> (refnum out=w272:refnum<file>, text=w269:string, error out=w273:errorcluster)  [unwired: 3 in, 1 out]
        n196 = Read from Text File(file (use dialog)=w287) -> (refnum out=w282:refnum<file>, text=w286:string, error out=w281:errorcluster)  [unwired: 3 in, 1 out]
        n197 = local read "riga sensore da modificare"() -> (w262:string)
        n198 = Unbundle By Name(w294) -> ("NOME"=w267:string, "Descrizione"=w264:string, "AI_min"=w293:dbl, "AI_max"=w292:dbl)
        n199 = Close File(refnum=w272, error in=w273) -> (path=w274:path, error out=w275:errorcluster)
        n200 = Close File(refnum=w282, error in=w281) -> (path=w280:path, error out=w279:errorcluster)
        n201 = Number To Fractional String(number=w293, precision (6)=w291) -> (F-format string=w260:string)  [unwired: 2 in]
        n202 = Number To Fractional String(number=w292, precision (6)=w291) -> (F-format string=w258:string)  [unwired: 2 in]
        n203 = Concatenate Strings(w267, w259, w264, w259, w260, w259, w258) -> (w257:string)
        n204 = Search and Replace String(replace all?=TRUE ("replace all? (F)"), input string=w269, search string=w262, replace string=w257, error in=w275) -> (result string=w271:string, error out=w276:errorcluster)  [unwired: 3 in, 2 out]
        n205 = Build Array(w267, w264, w260, w258) -> (w261:string[])
        n206 = Array Size(array=w261) -> (size(s)=w289:i32)
        n207 = Write to Text File(file (use dialog)=w274, text=w271, error in=w276) -> ()  [unwired: 1 in, 3 out]
        n208 = Decrement(x=w289) -> (x-1=w288:i32)
        n209 = for {
          shift-right: [w302] -> w285
          shift-left: "" ("format string") -> [w303]
          tunnel: w261 -> [w301] mode=indexing
          tunnel: w288 -> [w299]
          i -> [w300]
          n210 = Less?(x=w300, y=w299) -> (x < y?=w298:bool)
          n211 = Select(t="::" ("string"), s=w298, f="") -> (s? t:f=w295:string)
          n212 = Concatenate Strings(w303, w301, w295) -> (w302:string)
        }
        n213 = Search and Replace String(replace all?=TRUE ("replace all? (F)"), input string=w286, search string=w262, replace string=w285, error in=w279) -> (result string=w283:string, error out=w278:errorcluster)  [unwired: 3 in, 2 out]
        n214 = Write to Text File(file (use dialog)=w280, text=w283, error in=w278) -> ()  [unwired: 1 in, 3 out]
        n215 = property on="Salva modifica sensore" class="Bool"("Visible"=w277) -> ()  [unwired: 2 in, 2 out]
        n216 = property on="SENSORE SELEZIONATO" class="Clust (strict)"("Visible"=w277) -> ()  [unwired: 2 in, 2 out]
        n217 = property on="carica lista sensori" class="Bool (strict)"("Val(Sgnl)"=w266) -> (error out=w265:errorcluster)  [unwired: 2 in, 1 out]
        n218 = property on="carica mappatura" class="Bool (strict)"(error in=w265, "Val(Sgnl)"=w266) -> ()  [unwired: 1 in, 2 out]
      }
      event "modifica sensore": Value Change {
        w307 = "::" ("string")
        w311 = TRUE ("Visible")
        n219 = event-data() -> ()  [unwired: 1 in, 6 out]
        n220 = property on="Salva modifica sensore" class="Bool"("Visible"=w311) -> ()  [unwired: 2 in, 2 out]
        n221 = property on="SENSORE SELEZIONATO" class="Clust (strict)"("Visible"=w311) -> ()  [unwired: 2 in, 2 out]
        n222 = property on="LISTA SENSORI 2" class="MCListbox (strict)"() -> ("ItemNames"=w324:string[][], "Value"=w323:i32)  [unwired: 2 in, 2 out]
        n223 = Index Array(array=w324, index (row)=w323) -> (element=w315:string[])  [unwired: 1 in]
        n224 = Array Size(array=w315) -> (size(s)=w314:i32)
        n225 = Index Array(array=w315) -> (element #1=w310:string, element #2=w309:string, element #3=w320:string, element #4=w318:string)  [unwired: 6 in, 2 out]
        n226 = call-poly <vilib>:"Read Delimited Spreadsheet.vi"("file path (dialog if empty)"=w304, "delimiter (\\t)"="::" ("delimiter (\\t)")) -> ()  [unwired: 8 in, 6 out]
        n227 = Decrement(x=w314) -> (x-1=w312:i32)
        n228 = Concatenate Strings(w310, w307, w309, w307) -> (→"nome e desc sensore da modificare":string)
        n229 = call "String To Dbl.vi"("String"=w320) -> ("Numeric"=w319:dbl)  [unwired: 10 in]
        n230 = call "String To Dbl.vi"("String"=w318) -> ("Numeric"=w317:dbl)  [unwired: 10 in]
        n231 = for {
          shift-right: [w332] -> w313
          shift-left: "" ("format string") -> [w333]
          tunnel: w315 -> [w331] mode=indexing
          tunnel: w312 -> [w329]
          i -> [w330]
          n232 = Less?(x=w330, y=w329) -> (x < y?=w328:bool)
          n233 = Select(t="::" ("string"), s=w328, f="") -> (s? t:f=w325:string)
          n234 = Concatenate Strings(w333, w331, w325) -> (w332:string)
        }
        "riga sensore da modificare" <- w313
        n235 = Bundle By Name(cluster="SENSORE SELEZIONATO", "NOME"=w310, "Descrizione"=w309, "AI_min"=w319, "AI_max"=w317) -> (w321:T4)
        n236 = local write "SENSORE SELEZIONATO"(w321) -> ()
      }
      event "carica lista sensori": Value Change {
        n237 = event-data() -> ()  [unwired: 1 in, 6 out]
        n238 = call-poly <vilib>:"Read Delimited Spreadsheet.vi"("file path (dialog if empty)"=w338, "delimiter (\\t)"="::" ("delimiter (\\t)")) -> ("all rows"=w336:string[][])  [unwired: 8 in, 5 out]
        n239 = property on="LISTA SENSORI 2" class="MCListbox (strict)"("ItemNames"=w336) -> ()  [unwired: 2 in, 2 out]
        n240 = property on="LISTA SENSORI" class="MCListbox (strict)"("ItemNames"=w336) -> ()  [unwired: 2 in, 2 out]
        n241 = local write "aggiungi nuovo sensore"(FALSE ("aggiungi nuovo sensore")) -> ()
      }
      event "aggiungi nuovo sensore": Value Change {
        w347 = i16 3 ("precision (6)")
        n242 = event-data() -> ()  [unwired: 1 in, 6 out]
        n243 = property on="LISTA SENSORI 2" class="MCListbox (strict)"() -> ("ItemNames"=w342:string[][])  [unwired: 2 in, 2 out]
        n244 = Unbundle By Name("NUOVO SENSORE") -> ("NOME"=w346:string, "Descrizione"=w345:string, "AI_min"=w349:dbl, "AI_max"=w348:dbl)
        n245 = Number To Fractional String(number=w349, precision (6)=w347) -> (F-format string=w344:string)  [unwired: 2 in]
        n246 = Number To Fractional String(number=w348, precision (6)=w347) -> (F-format string=w343:string)  [unwired: 2 in]
        n247 = Build Array(w346, w345, w344, w343) -> (w341:string[])
        n248 = Build Array (concatenate)(w342, w341) -> (w340:string[][])
        n249 = property on="LISTA SENSORI 2" class="MCListbox (strict)"("ItemNames"=w340) -> ()  [unwired: 2 in, 2 out]
      }
      event "ELIMINA SENSORE": Value Change {
        n250 = event-data() -> ()  [unwired: 1 in, 6 out]
        n251 = Two Button Dialog(message="ELIMINARE IL SENSORE SELEZIONATO?\n\nLa mappatura ingressi-sensori verrà\naggiornata di conseguenza.") -> (T button?=w353:bool)  [unwired: 2 in]
        n252 = case shown="True" w353 {
          tunnel: w352 -> [_ w364]
          frame False {
          }
          frame True {
            n253 = property on="LISTA SENSORI 2" class="MCListbox (strict)"() -> ("ItemNames"=w367:string[][], "Value"=w366:i32)  [unwired: 2 in, 2 out]
            n254 = call-poly <vilib>:"Read Delimited Spreadsheet.vi"("file path (dialog if empty)"=w364, "delimiter (\\t)"="::" ("delimiter (\\t)")) -> ("new file path (Not A Path if cancelled)"=w358:path, "all rows"=w363:string[][])  [unwired: 8 in, 4 out]
            n255 = Delete From Array(array=w367, index (row)=w366) -> (deleted portion=w361:string[], array with subset deleted=w362:string[][])  [unwired: 2 in]
            n256 = Index Array(array=w361, index=0 ("disabled index (col)")) -> (element=w359:string)
            n257 = property on="LISTA SENSORI 2" class="MCListbox (strict)"("ItemNames"=w362) -> ()  [unwired: 2 in, 2 out]
            n258 = for {
              tunnel: w363 -> [w369] mode=indexing
              tunnel: w359 -> [w370]
              tunnel: [w369] -> w357 mode=indexing if=w368
              n259 = Index Array(array=w369, index=1) -> (element=w371:string)
              n260 = Not Equal?(x=w370, y=w371) -> (x != y?=w368:bool)
            }
            n261 = property on="carica mappatura" class="Bool (strict)"("Val(Sgnl)"=TRUE ("Value (Signaling)")) -> ()  [unwired: 2 in, 2 out]
            n262 = call-poly <vilib>:"Write Delimited Spreadsheet.vi"("file path (dialog if empty)"=w358, "2D data"=w357, "delimiter (\\t)"="::" ("delimiter (\\t)")) -> ()  [unwired: 11 in, 2 out]
          }
        }
      }
      event "stop": Value Change; Panel Close {
        n263 = event-data() -> ()  [unwired: 1 in, 3 out]
      }
      event "Associa sensore": Value Change {
        n264 = event-data() -> ()  [unwired: 1 in, 6 out]
        n265 = disable-structure shown="Enabled" {
          frame Disabled {
            n266 = property on="LISTA SENSORI ASSOCIATI" class="MCListbox (strict)"() -> ("ItemNames"=w383:string[][], "Value"=w382:i32)  [unwired: 2 in, 2 out]
            n267 = property on="LISTA SENSORI" class="MCListbox (strict)"() -> ("Value"=w385:i32, "ItemNames"=w386:string[][])  [unwired: 2 in, 2 out]
            n268 = Index Array(array=w386, index (row)=w385, index (col)=0 ("disabled index (col)")) -> (element=w380:string)
            n269 = Index Array(array=w383, index (row)=w382) -> (element=w378:string[])  [unwired: 1 in]
            n270 = Search 1D Array(1D array=w378, element="") -> (index of element=w376:i32)  [unwired: 1 in]
            n271 = Replace Array Subset(array=w378, new element=w380, index=w376) -> (w379:string[])
            n272 = Replace Array Subset(array=w383, new element=w379, index (row)=w382) -> (w381:string[][])  [unwired: 1 in]
            n273 = property on="LISTA SENSORI ASSOCIATI" class="MCListbox (strict)"("ItemNames"=w381) -> ()  [unwired: 2 in, 2 out]
          }
          frame Enabled {
            n274 = property on="LISTA INGRESSI 3" class="MCListbox (strict)"() -> ("Value"=w394:i32, "ItemNames"=w395:string[][])  [unwired: 2 in, 2 out]
            n275 = property on="LISTA SENSORI" class="MCListbox (strict)"() -> ("Value"=w393:i32, "ItemNames"=w402:string[][])  [unwired: 2 in, 2 out]
            n276 = Index Array(array=w402, index (row) #1=w393, index (col) #1=0 ("disabled index (col)"), index (row) #2=w393) -> (element #1=w397:string, element #2=w392:string[])  [unwired: 1 in]
            n277 = Index Array(array=w395, index (row)=w394, index (col)=0 ("disabled index (col)")) -> (element=w398:string)
            n278 = Array Subset(array=w392, index=1 ("index (row)")) -> (w390:string[])  [unwired: 1 in]
            n279 = property on="MAPPATURA" class="Tbl (strict)"() -> ("Value"=w400:string[][])  [unwired: 2 in, 2 out]
            n280 = Build Array (concatenate)(w398, w397, w390, string[] ["", "", ""], "ASSENTE", "RANGE/OFFSET") -> (w396:string[])
            n281 = Insert Into Array(array=w400, new element=w396) -> (w399:string[][])  [unwired: 2 in]
            n282 = property on="MAPPATURA" class="Tbl (strict)"("Value"=w399) -> ()  [unwired: 2 in, 2 out]
          }
        }
      }
      event "Elimina sensori ingresso selezionato": Value Change {
        n283 = event-data() -> ()  [unwired: 1 in, 6 out]
        n284 = disable-structure shown="Enabled" {
          frame Disabled {
            w410 = "" ("element")
            n285 = property on="LISTA SENSORI ASSOCIATI" class="MCListbox (strict)"() -> ("ItemNames"=w409:string[][], "Value"=w408:i32)  [unwired: 2 in, 2 out]
            n286 = Index Array(array=w409, index (row)=w408) -> (element=w412:string[])  [unwired: 1 in]
            n287 = Index Array(array=w412) -> (element=w411:string)  [unwired: 1 in]
            n288 = Build Array(w411, w410, w410, w410, w410, w410) -> (w407:string[])
            n289 = Replace Array Subset(array=w409, new element=w407, index (row)=w408) -> (w406:string[][])  [unwired: 1 in]
            n290 = property on="LISTA SENSORI ASSOCIATI" class="MCListbox (strict)"("ItemNames"=w406) -> ()  [unwired: 2 in, 2 out]
          }
          frame Enabled {
            n291 = property on="MAPPATURA" class="Tbl (strict)" props=["Value", "Active Cell"]() -> ("Value"=w416:string[][])  [unwired: 2 in, 3 out]
            n292 = property on="Edit Position" class="Clust (strict)"() -> ("Value"=w414:T1)  [unwired: 2 in, 2 out]
            n293 = Unbundle By Name(w414) -> ("Row"=w413:i32)
            n294 = Delete From Array(array=w416, index (row)=w413) -> (array with subset deleted=w415:string[][])  [unwired: 2 in, 1 out]
            n295 = property on="MAPPATURA" class="Tbl (strict)"("Value"=w415) -> ()  [unwired: 2 in, 2 out]
          }
        }
        n296 = local write "Elimina sensori ingresso selezionato"(FALSE ("Elimina sensori ingresso selezionato")) -> ()
      }
      event "Salva mappatura ingressi sensori": Value Change {
        n297 = event-data() -> ()  [unwired: 1 in, 6 out]
        n298 = property on="MAPPATURA" class="Tbl (strict)"() -> ("Value"=w419:string[][])  [unwired: 2 in, 2 out]
        n299 = call-poly <vilib>:"Write Delimited Spreadsheet.vi"("file path (dialog if empty)"=w421, "2D data"=w419, "delimiter (\\t)"="::" ("delimiter (\\t)")) -> ()  [unwired: 11 in, 2 out]
        n300 = property on="Salva mappatura ingressi sensori" class="Bool (strict)"("Value"=FALSE ("Salva mappatura ingressi sensori")) -> ()  [unwired: 2 in, 2 out]
      }
      event "carica mappatura": Value Change {
        n301 = event-data() -> ()  [unwired: 1 in, 6 out]
        n302 = call-poly <vilib>:"Read Delimited Spreadsheet.vi"("file path (dialog if empty)"=w427, "delimiter (\\t)"="::" ("delimiter (\\t)")) -> ("all rows"=w425:string[][])  [unwired: 8 in, 5 out]
        n303 = for {
          tunnel: w425 -> [w447] mode=indexing
          tunnel: [w443] -> w424 mode=indexing
          w431 = "FUNZ. CORR." ("y")
          w437 = "PRESENTE" ("y")
          n304 = Initialize Array("", 31 ("dimension size")) -> (w444:string[])
          n305 = Replace Array Subset "Replace Array Subset"(array=w444, new element=w447) -> (w441:string[])  [unwired: 1 in]
          n306 = Index Array(array=w441, index #1=8 ("index"), index #2=9 ("index")) -> (element #1=w439:string, element #2=w429:string)
          n307 = Equal?(x=w429, y=w431) -> (x = y?=w430:bool)
          n308 = Equal?(x=w439, y=w437) -> (x = y?=w438:bool)
          n309 = Select(t=w431, s=w430, f="RANGE/OFFSET" ("y")) -> (s? t:f=w428:string)
          n310 = Select(t=w437, s=w438, f="ASSENTE" ("y")) -> (s? t:f=w435:string)
          n311 = Replace Array Subset(array=w441, new element #1=w435, index #1=8 ("index"), new element #2=w428, index #2=9 ("index")) -> (w443:string[])
        }
        n312 = local write "carica mappatura"(FALSE ("carica mappatura")) -> ()
        n313 = property on="MAPPATURA" class="Tbl (strict)"("Value"=w424) -> ()  [unwired: 2 in, 2 out]
      }
      event "MAPPATURA": Mouse Up {
        n314 = event-data() -> ()  [unwired: 1 in, 8 out]
        n315 = property on="MAPPATURA" class="Tbl (strict)"() -> ("EditPos"=w449:T1, "Value"=w453:string[][])  [unwired: 2 in, 2 out]
        "Edit Position" <- w449
        n316 = Unbundle By Name(w449) -> ("Column"=w451:i32)
        n317 = Equal?(x=w451, y=7) -> (x = y?=w454:bool)
        n318 = Equal?(x=w451, y=8) -> (x = y?=w450:bool)
        n319 = case shown="True" w450 {
          tunnel: w449 -> [_ w474]
          frame False {
          }
          frame True {
            n320 = property on="MAPPATURA" class="Tbl (strict)"() -> ("Value"=w471:string[][])  [unwired: 2 in, 2 out]
            n321 = Unbundle By Name(w474) -> ("Row"=w470:i32)  [unwired: 1 out]
            n322 = Index Array(array=w471, index (row)=w470) -> (element=w462:string[])  [unwired: 1 in]
            n323 = Array Subset(array=w462, index=11, length=20) -> (w466:string[])
            n324 = Index Array(array=w462, index #1=9 ("index")) -> (element #1=w460:string, element #2=w457:string)  [unwired: 1 in]
            n325 = Array Size(array=w466) -> (size(s)=w465:i32)
            n326 = Decimal String To Number(string=w457) -> (number=w456:i32)  [unwired: 2 in, 1 out]
            n327 = Divide(x=w465, y=2) -> (x/y=w463:dbl)
            n328 = for {
              N: w463 -> [_]
              shift-right: [w478] -> _
              shift-left: w466 -> [w481]
              tunnel: [w476] -> w467 mode=indexing if=w475
              n329 = Delete From Array(array=w481, length=2, index=0) -> (deleted portion=w476:string[], array with subset deleted=w478:string[])
              n330 = Not Equal?(x=w476, y=string[] ["", ""] ("deleted portion")) -> (x != y?=w475:bool)
            }
            n331 = Equal?(x=w460, y="1") -> (x = y?=w458:bool)
            n332 = property on="USA FUNZIONE CORRETTRICE?" class="Bool (strict)"("Value"=w458) -> ()  [unwired: 2 in, 2 out]
            n333 = property on="Ordine polinomio fit" class="DigNum (strict)"("Value"=w456) -> ()  [unwired: 2 in, 2 out]
            n334 = property on="PUNTI FUNZIONE CORRETTRICE" class="MCListbox (strict)"("ItemNames"=w467) -> ()  [unwired: 2 in, 2 out]
            n335 = property on="MAPPATURA" class="Tbl (strict)"("DisabledEnum"=T6."Disabled and Grayed Out" ("Disabled")) -> ()  [unwired: 2 in, 2 out]
            n336 = property on="Cluster Funzione correttrice" class="Clust"("Visible"=TRUE) -> ()  [unwired: 2 in, 2 out]
          }
        }
        n337 = case shown="True" w454 {
          tunnel: w453 -> [_ w487]
          tunnel: w449 -> [_ w486]
          frame False {
          }
          frame True {
            n338 = call "UM.vi"() -> ("annulla?"=w482:bool, "RingText.Text"=w483:string)  [unwired: 10 in]
            n339 = Unbundle By Name(w486) -> ("Row"=w485:i32, "Column"=w484:i32)
            n340 = case shown="False" w482 {
              tunnel: w487 -> [w492 _]
              tunnel: w485 -> [w491 _]
              tunnel: w484 -> [w490 _]
              tunnel: w483 -> [w488 _]
              frame False {
                n341 = Replace Array Subset(array=w492, new element=w488, index (row)=w491, index (col)=w490) -> (w489:string[][])
                n342 = property on="MAPPATURA" class="Tbl (strict)"("Value"=w489) -> ()  [unwired: 2 in, 2 out]
              }
              frame True {
              }
            }
          }
        }
      }
      event "MANAGER FUNZIONE CORRETTRICE": Value Change {
        n343 = event-data() -> ("NewVal"=w494:bool)  [unwired: 1 in, 5 out]
        n344 = case shown="True" w494 {
          frame False {
          }
          frame True {
            n345 = property on="MAPPATURA" class="Tbl (strict)"() -> ("Value"=w511:string[][])  [unwired: 2 in, 2 out]
            n346 = local read "Row"() -> (w496:i32)
            n347 = Index Array(array=w511, index (row)=w496) -> (element=w503:string[])  [unwired: 1 in]
            n348 = Array Subset(array=w503, index=11, length=20) -> (w507:string[])
            n349 = Index Array(array=w503, index #1=9 ("index")) -> (element #1=w501:string, element #2=w498:string)  [unwired: 1 in]
            n350 = Array Size(array=w507) -> (size(s)=w506:i32)
            n351 = Decimal String To Number(string=w498) -> (number=w497:i32)  [unwired: 2 in, 1 out]
            n352 = Divide(x=w506, y=2) -> (x/y=w504:dbl)
            n353 = for {
              N: w504 -> [_]
              shift-right: [w517] -> _
              shift-left: w507 -> [w520]
              tunnel: [w515] -> w508 mode=indexing if=w514
              n354 = Delete From Array(array=w520, length=2, index=0) -> (deleted portion=w515:string[], array with subset deleted=w517:string[])
              n355 = Not Equal?(x=w515, y=string[] ["", ""] ("deleted portion")) -> (x != y?=w514:bool)
            }
            n356 = Equal?(x=w501, y="FUNZ. CORR.") -> (x = y?=w499:bool)
            n357 = property on="USA FUNZIONE CORRETTRICE?" class="Bool (strict)"("Value"=w499) -> ()  [unwired: 2 in, 2 out]
            n358 = property on="Ordine polinomio fit" class="DigNum (strict)"("Value"=w497) -> ()  [unwired: 2 in, 2 out]
            n359 = property on="PUNTI FUNZIONE CORRETTRICE" class="MCListbox (strict)"("ItemNames"=w508) -> ()  [unwired: 2 in, 2 out]
            n360 = property on="MAPPATURA" class="Tbl (strict)"("DisabledEnum"=T6."Disabled and Grayed Out" ("Disabled")) -> ()  [unwired: 2 in, 2 out]
            n361 = property on="Cluster Funzione correttrice" class="Clust"("Visible"=TRUE) -> ()  [unwired: 2 in, 2 out]
          }
        }
        n362 = local write "MANAGER FUNZIONE CORRETTRICE"(FALSE ("MANAGER FUNZIONE CORRETTRICE")) -> ()
      }
      event "MAPPATURA": Mouse Down {
        # "The row clicked on last time:\nchange the background color back to blank"
        n363 = event-data() -> ()  [unwired: 1 in, 8 out]
        n364 = property on="MAPPATURA" class="Tbl (strict)"() -> ("Selection Start"=w523:T1)  [unwired: 2 in, 2 out]
        n365 = property on="MAPPATURA" class="Tbl (strict)"() -> ("Number of Columns"=w524:u32)  [unwired: 2 in, 2 out]
        n366 = Unbundle By Name(w522) -> ("Row"=w526:i32)  [unwired: 1 out]
        n367 = Unbundle By Name(w523) -> ("Row"=w521:i32)  [unwired: 1 out]
        "Row" <- w521
        n368 = for {
          N: w524 -> [_]
          tunnel: u32 16448250 -> [w528]
          tunnel: w522 -> [w532]
          tunnel: w526 -> [w531]
          i -> [w530]
          n369 = Bundle(cluster=w532, "Row"=w531, "Column"=w530) -> (w529:T1)
          n370 = property on="MAPPATURA" class="Tbl (strict)"("Active Cell"=w529, "Cell BG Color"=w528) -> ()  [unwired: 2 in, 2 out]
        }
        n371 = for {
          N: w524 -> [_]
          tunnel: u32 14483200 -> [w533]
          tunnel: w523 -> [w537]
          tunnel: w521 -> [w536]
          i -> [w535]
          n372 = Bundle(cluster=w537, "Row"=w536, "Column"=w535) -> (w534:T1)
          n373 = property on="MAPPATURA" class="Tbl (strict)"("Active Cell"=w534, "Cell BG Color"=w533) -> ()  [unwired: 2 in, 2 out]
        }
      }
      event "SALVA ASSOC INGRESSI-LINEE": Value Change {
        n374 = event-data() -> ()  [unwired: 1 in, 6 out]
        n375 = control-ref of="LINEA 1 - PORTATA"() -> (w567:refnum<vi>)
        n376 = control-ref of="LINEA 1 - PRESSIONE MANDATA"() -> (w565:refnum<vi>)
        n377 = control-ref of="LINEA 1 - PRESSIONE ASPIRAZIONE"() -> (w564:refnum<vi>)
        n378 = control-ref of="LINEA 1 - PRESSIONE PREMISTOPPA"() -> (w549:refnum<vi>)
        n379 = control-ref of="LINEA 1 - COPPIA"() -> (w542:refnum<vi>)
        n380 = control-ref of="LINEA 2 - PORTATA"() -> (w544:refnum<vi>)
        n381 = control-ref of="LINEA 2 - PRESSIONE MANDATA"() -> (w563:refnum<vi>)
        n382 = control-ref of="LINEA 2 - PRESSIONE ASPIRAZIONE"() -> (w562:refnum<vi>)
        n383 = control-ref of="LINEA 2 - PRESSIONE PREMISTOPPA"() -> (w548:refnum<vi>)
        n384 = control-ref of="LINEA 2 - COPPIA"() -> (w541:refnum<vi>)
        n385 = control-ref of="LINEA 3 - PORTATA"() -> (w561:refnum<vi>)
        n386 = control-ref of="LINEA 3 - PRESSIONE MANDATA"() -> (w560:refnum<vi>)
        n387 = control-ref of="LINEA 3 - PRESSIONE ASPIRAZIONE"() -> (w559:refnum<vi>)
        n388 = control-ref of="LINEA 3 - PRESSIONE PREMISTOPPA"() -> (w547:refnum<vi>)
        n389 = control-ref of="LINEA 3 - COPPIA"() -> (w540:refnum<vi>)
        n390 = control-ref of="LINEA 4 - PORTATA"() -> (w556:refnum<vi>)
        n391 = control-ref of="LINEA 4 - PRESSIONE MANDATA"() -> (w555:refnum<vi>)
        n392 = control-ref of="LINEA 4 - PRESSIONE ASPIRAZIONE"() -> (w554:refnum<vi>)
        n393 = control-ref of="LINEA 4 - PRESSIONE PREMISTOPPA"() -> (w546:refnum<vi>)
        n394 = control-ref of="LINEA 4 - COPPIA"() -> (w539:refnum<vi>)
        n395 = control-ref of="LINEA 5 - PORTATA"() -> (w553:refnum<vi>)
        n396 = control-ref of="LINEA 5 - PRESSIONE MANDATA"() -> (w552:refnum<vi>)
        n397 = control-ref of="LINEA 5 - PRESSIONE ASPIRAZIONE"() -> (w551:refnum<vi>)
        n398 = control-ref of="LINEA 5 - PRESSIONE PREMISTOPPA"() -> (w545:refnum<vi>)
        n399 = control-ref of="LINEA 5 - COPPIA"() -> (w538:refnum<vi>)
        n400 = Build Array(w567, w565, w564, w549, w542, w544, w563, w562, w548, w541, w561, w560, w559, w547, w540, w556, w555, w554, w546, w539, w553, w552, w551, w545, w538) -> (w566:refnum<vi>[])
        n401 = for {
          tunnel: w566 -> [w573] mode=indexing
          tunnel: [w568] -> w543 mode=indexing
          n402 = property class="MCListbox (strict)"(reference=w573) -> ("Label.Text"=w569:string, "ItemNames"=w572:string[][])  [unwired: 1 in, 2 out]
          n403 = Index Array(array=w572, index (col)=0 ("disabled index (col)")) -> (element=w570:string[])  [unwired: 1 in]
          n404 = Build Array (concatenate)(w569, w570) -> (w568:string[])
        }
        n405 = call-poly <vilib>:"Write Delimited Spreadsheet.vi"("file path (dialog if empty)"=w557, "2D data"=w543, "delimiter (\\t)"="::" ("delimiter (\\t)")) -> ()  [unwired: 11 in, 2 out]
      }
      event "carica assoc ingressi- linee": Value Change {
        n406 = event-data() -> ()  [unwired: 1 in, 6 out]
        n407 = control-ref of="LINEA 1 - PORTATA"() -> (w599:refnum<vi>)
        n408 = control-ref of="LINEA 1 - PRESSIONE MANDATA"() -> (w598:refnum<vi>)
        n409 = control-ref of="LINEA 1 - PRESSIONE ASPIRAZIONE"() -> (w597:refnum<vi>)
        n410 = control-ref of="LINEA 1 - PRESSIONE PREMISTOPPA"() -> (w585:refnum<vi>)
        n411 = control-ref of="LINEA 1 - COPPIA"() -> (w579:refnum<vi>)
        n412 = control-ref of="LINEA 2 - PORTATA"() -> (w580:refnum<vi>)
        n413 = control-ref of="LINEA 2 - PRESSIONE MANDATA"() -> (w596:refnum<vi>)
        n414 = control-ref of="LINEA 2 - PRESSIONE ASPIRAZIONE"() -> (w595:refnum<vi>)
        n415 = control-ref of="LINEA 2 - PRESSIONE PREMISTOPPA"() -> (w584:refnum<vi>)
        n416 = control-ref of="LINEA 2 - COPPIA"() -> (w578:refnum<vi>)
        n417 = control-ref of="LINEA 3 - PORTATA"() -> (w594:refnum<vi>)
        n418 = control-ref of="LINEA 3 - PRESSIONE MANDATA"() -> (w593:refnum<vi>)
        n419 = control-ref of="LINEA 3 - PRESSIONE ASPIRAZIONE"() -> (w592:refnum<vi>)
        n420 = control-ref of="LINEA 3 - PRESSIONE PREMISTOPPA"() -> (w583:refnum<vi>)
        n421 = control-ref of="LINEA 3 - COPPIA"() -> (w577:refnum<vi>)
        n422 = control-ref of="LINEA 4 - PORTATA"() -> (w591:refnum<vi>)
        n423 = control-ref of="LINEA 4 - PRESSIONE MANDATA"() -> (w590:refnum<vi>)
        n424 = control-ref of="LINEA 4 - PRESSIONE ASPIRAZIONE"() -> (w589:refnum<vi>)
        n425 = control-ref of="LINEA 4 - PRESSIONE PREMISTOPPA"() -> (w582:refnum<vi>)
        n426 = control-ref of="LINEA 4 - COPPIA"() -> (w576:refnum<vi>)
        n427 = control-ref of="LINEA 5 - PORTATA"() -> (w588:refnum<vi>)
        n428 = control-ref of="LINEA 5 - PRESSIONE MANDATA"() -> (w587:refnum<vi>)
        n429 = control-ref of="LINEA 5 - PRESSIONE ASPIRAZIONE"() -> (w586:refnum<vi>)
        n430 = control-ref of="LINEA 5 - PRESSIONE PREMISTOPPA"() -> (w581:refnum<vi>)
        n431 = control-ref of="LINEA 5 - COPPIA"() -> (w575:refnum<vi>)
        n432 = Build Array(w599, w598, w597, w585, w579, w580, w596, w595, w584, w578, w594, w593, w592, w583, w577, w591, w590, w589, w582, w576, w588, w587, w586, w581, w575) -> (w574:refnum<vi>[])
        n433 = call-poly <vilib>:"Read Delimited Spreadsheet.vi"("file path (dialog if empty)"=w602, "delimiter (\\t)"="::" ("delimiter (\\t)")) -> ("all rows"=w601:string[][])  [unwired: 8 in, 5 out]
        n434 = for {
          tunnel: w574 -> [w607] mode=indexing
          tunnel: w601 -> [w610] mode=indexing
          n435 = Delete From Array(array=w610, length=1, index=0) -> (array with subset deleted=w606:string[])  [unwired: 1 out]
          n436 = Build Array(w606) -> (w605:string[][])
          n437 = Transpose 2D Array(2D array=w605) -> (transposed array=w604:string[][])
          n438 = property class="MCListbox (strict)"(reference=w607, "ItemNames"=w604) -> ()  [unwired: 1 in, 2 out]
        }
      }
      event "SVUOTA TUTTO MAPPATURA": Value Change {
        n439 = event-data() -> ()  [unwired: 1 in, 6 out]
        n440 = control-ref of="LINEA 1 - PORTATA"() -> (w636:refnum<vi>)
        n441 = control-ref of="LINEA 1 - PRESSIONE MANDATA"() -> (w635:refnum<vi>)
        n442 = control-ref of="LINEA 1 - PRESSIONE ASPIRAZIONE"() -> (w634:refnum<vi>)
        n443 = control-ref of="LINEA 1 - PRESSIONE PREMISTOPPA"() -> (w622:refnum<vi>)
        n444 = control-ref of="LINEA 1 - COPPIA"() -> (w616:refnum<vi>)
        n445 = control-ref of="LINEA 2 - PORTATA"() -> (w617:refnum<vi>)
        n446 = control-ref of="LINEA 2 - PRESSIONE MANDATA"() -> (w633:refnum<vi>)
        n447 = control-ref of="LINEA 2 - PRESSIONE ASPIRAZIONE"() -> (w632:refnum<vi>)
        n448 = control-ref of="LINEA 2 - PRESSIONE PREMISTOPPA"() -> (w621:refnum<vi>)
        n449 = control-ref of="LINEA 2 - COPPIA"() -> (w615:refnum<vi>)
        n450 = control-ref of="LINEA 3 - PORTATA"() -> (w631:refnum<vi>)
        n451 = control-ref of="LINEA 3 - PRESSIONE MANDATA"() -> (w630:refnum<vi>)
        n452 = control-ref of="LINEA 3 - PRESSIONE ASPIRAZIONE"() -> (w629:refnum<vi>)
        n453 = control-ref of="LINEA 3 - PRESSIONE PREMISTOPPA"() -> (w620:refnum<vi>)
        n454 = control-ref of="LINEA 3 - COPPIA"() -> (w614:refnum<vi>)
        n455 = control-ref of="LINEA 4 - PORTATA"() -> (w628:refnum<vi>)
        n456 = control-ref of="LINEA 4 - PRESSIONE MANDATA"() -> (w627:refnum<vi>)
        n457 = control-ref of="LINEA 4 - PRESSIONE ASPIRAZIONE"() -> (w626:refnum<vi>)
        n458 = control-ref of="LINEA 4 - PRESSIONE PREMISTOPPA"() -> (w619:refnum<vi>)
        n459 = control-ref of="LINEA 4 - COPPIA"() -> (w613:refnum<vi>)
        n460 = control-ref of="LINEA 5 - PORTATA"() -> (w625:refnum<vi>)
        n461 = control-ref of="LINEA 5 - PRESSIONE MANDATA"() -> (w624:refnum<vi>)
        n462 = control-ref of="LINEA 5 - PRESSIONE ASPIRAZIONE"() -> (w623:refnum<vi>)
        n463 = control-ref of="LINEA 5 - PRESSIONE PREMISTOPPA"() -> (w618:refnum<vi>)
        n464 = control-ref of="LINEA 5 - COPPIA"() -> (w612:refnum<vi>)
        n465 = Build Array(w636, w635, w634, w622, w616, w617, w633, w632, w621, w615, w631, w630, w629, w620, w614, w628, w627, w626, w619, w613, w625, w624, w623, w618, w612) -> (w611:refnum<vi>[])
        n466 = for {
          tunnel: w611 -> [w639] mode=indexing
          n467 = property class="MCListbox (strict)"(reference=w639, "ItemNames"=string[][] [] ("Item Names")) -> ()  [unwired: 1 in, 2 out]
        }
      }
    }
  }
  n468 = for {
    tunnel: w17 -> [w641] mode=indexing
    n469 = property class="MCListbox (strict)"(reference=w641, "ItemNames"=string[][] [] ("Item Names")) -> ()  [unwired: 1 in, 2 out]
  }
